vi "agilent test 13.0 Final.vi"() -> ()   [LabVIEW 2023]
uses:
  <vilib>/Utility/file.llb/Write Delimited Spreadsheet (string).vi
  <vilib>/Utility/file.llb/Write Delimited Spreadsheet (DBL).vi
  <vilib>/express/express arith-compare/Formula/XNode/ExpressFormulaBlockNode.xnode
panel:
  in  "Stop running transfer characteristics":bool
  in  "stop OUTPUT":bool
  out "dID":dbl
  in  "SIM VG OUT":dbl[](array[numeric])
  in  "VG OC MEA":dbl[](array[numeric])
  in  "Mobility trans":dbl[](array[numeric])
  in  "IS OUTPUT":dbl[](array[numeric])
  in  "IG OUTPUT":dbl[](array[numeric])
  in  "ID OUTPUT":dbl[](array[numeric])
  in  "VD OUTPUT":dbl[](array[numeric])
  in  "IG TRANSFER":dbl[](array[numeric])
  in  "IS TRANSFER":dbl[](array[numeric])
  in  "ID TRANSFER":dbl[](array[numeric])
  in  "VG TRANSFER":dbl[](array[numeric])
  in  "state":dbl
  in  "output number of times":dbl
  in  "output TEM":dbl
  in  "IDS 6":dbl[](array[numeric])
  in  "IDS 5":dbl[](array[numeric])
  in  "IDS 4":dbl[](array[numeric])
  in  "IDS 3":dbl[](array[numeric])
  in  "IDS 2":dbl[](array[numeric])
  in  "IDS 1":dbl[](array[numeric])
  in  "VDS":dbl[](array[numeric])
  in  "transfer number of times":dbl
  in  "transfer Tem":dbl
  in  "IDS":dbl[](array[numeric])
  in  "VG":dbl[](array[numeric])
  in  "Characterization of TFT":enum32{"Simulation", " Transfer", "Output"}(tab)=enum." Transfer"
  in  "Clear":bool
  in  "Predicted mobility [cm^2/Vs] for OC":dbl
  out "Output characteristic simulation":cluster{"Value":dbl[], "Value":dbl[]}[](graph)
  in  "RUN OUTPUT":bool
  in  "VGS[5] [V] for OC":dbl
  in  "VGS[4] [V] for OC":dbl
  in  "VGS[3] [V] for OC":dbl
  in  "VGS[2] [V] for OC":dbl
  in  "VT [V] for OC":dbl
  in  "VGS[1] [V] for OC":dbl
  in  "Step for VDS [V] for OC":dbl
  in  "Transistor capacitance [nF/cm^2] for OC":dbl
  in  "Transistor length [cm] for OC":dbl
  in  "Transistor width [cm] for OC":dbl
  out "Transfer characteristic simulation":cluster{"Y":dbl[], "Y":dbl[]}[](graph)
  in  "Predicted mobility [cm^2/Vs] for TC":dbl
  in  "Step for VGS [V] for TC":dbl
  in  "Maximum VDS [V] for OC":dbl
  in  "VT [V] for TC":dbl
  in  "VGS [V] for TC":dbl
  in  "Transistor capacitance [nF/cm^2] for TC":dbl
  in  "Transistor width [cm] for TC":dbl
  in  "Transistor length [cm] for TC":dbl
  in  "run":bool
  in  "VG[6] [V] for OC":dbl
  in  "Number of time of hysteresis (TC)":dbl=1.0
  in  "Sample(TC)":dbl=1.0
  out "Mobility":cluster{"Y":dbl[], "Y":dbl[]}[](graph)
  in  "Saturation":bool
  out "Mobility [cm^2/Vs]":dbl
  in  "Hysteresis(TC)":bool
  out "IG/VG":cluster{"Y":dbl[], "Y":dbl[]}[](graph)
  in  "integration(TC)":dbl=1.0
  out "IS/VG":cluster{"Y":dbl[], "Y":dbl[]}[](graph)
  out "ID/VG":cluster{"Y":dbl[], "Y":dbl[]}[](graph)
  out "ID [A](TC)":dbl
  out "IS [A](TC)":dbl
  out "IG [A](TC)":dbl
  in  "Run transfer":bool
  in  "VG Compliance(TC) [A]":dbl=0.001
  in  "VG SMU (T)":dbl=1.0
  in  "VG [V] Step(TC)":dbl=0.01
  in  "VG [V] Stop(TC)":dbl=2.2
  in  "VG [V] Start(TC)":dbl
  in  "VD Compliance(TC) [A] Compliance(TC)":dbl=0.001
  in  "VD SMU (T)":dbl=2.0
  in  "VD [V](TC)":dbl=2.2
  in  "VS Compliance(TC) [A]":dbl=0.001
  in  "VS SMU (T)":dbl=3.0
  in  "VS [V](TC)":dbl
  in  "VISA resource name(TC)":refnum<visa-resource-name>="GPIB0::16::INSTR"
  out "Current VG [V](TC)":dbl
  in  "Length [um]":dbl=10.0
  in  "Thickness [cm]":dbl=3e-07
  in  "Width [um]":dbl=1000.0
  in  "Number of time of hysteresis (OC)":dbl=1.0
  out "VG Measurement number":dbl
  out "VD Measurement number":dbl
  in  "Sample(OC)":dbl=1.0
  out "Current VG [V](OC)":dbl
  in  "Hysteresis(OC)":bool
  out "IG/VD":cluster{"Y":dbl[], "Y":dbl[]}[](graph)
  out "IS/VD":cluster{"Y":dbl[], "Y":dbl[]}[](graph)
  out "ID/VD":cluster{"Y":dbl[], "Y":dbl[]}[](graph)
  out "ID [A](OC)":dbl
  out "IS [A](OC)":dbl
  out "IG [A](OC)":dbl
  in  "VG Compliance(OC) [A]":dbl=0.001
  in  "VG SMU(OC)":dbl=1.0
  out "Current VD [V](OC)":dbl
  in  "VG [V] Step(OC)":dbl=0.4
  in  "VG [V] Stop(OC)":dbl=2.0
  in  "VG [V] Start(OC)":dbl
  in  "VD Compliance(OC) [A]":dbl=0.001
  in  "VD SMU(OC)":dbl=3.0
  in  "VD [V] Step(OC)":dbl=0.01
  in  "VD [V] Stop(OC)":dbl=2.0
  in  "VD [V] Start(OC)":dbl
  in  "VS Compliance(OC) [A]":dbl=0.001
  in  "VS SMU(OC)":dbl=2.0
  in  "VS [V](OC)":dbl
  in  "integration(OC)":dbl=1.0
  in  "RUN OUTPUT":bool
  in  "VISA resource name(OC)":refnum<visa-resource-name>="GPIB0::16::INSTR"
  # "Variables used in program"
  # "Transfer characteristics(TC)"
  # "Please set values below for transfer characteristic simulation"
  # "Run transfer characteristic simulation"
  # "When saving data to file, use .csv as extension filename."
  # "------------------------------------------------------------------------------------------------------------------------------------------------------------------------------------------------------------------------------------------------------------------------------------------------"
  # "Output characteristics(OC)"
  # "Please set values below for output characteristic simulation"
  # "Run output characteristic simulation"
  # "Please press clear to clear data and graph after each run."
  # "This can avoid lag of program"
  # "Clear both graph"
  # "TC stands for transfer characterization"
  # "Linear"
  # "When saving data to file, use .csv as extension filename."
  # "OC stands for output characterization"
  # "When saving data to file, use .csv as extension filename."
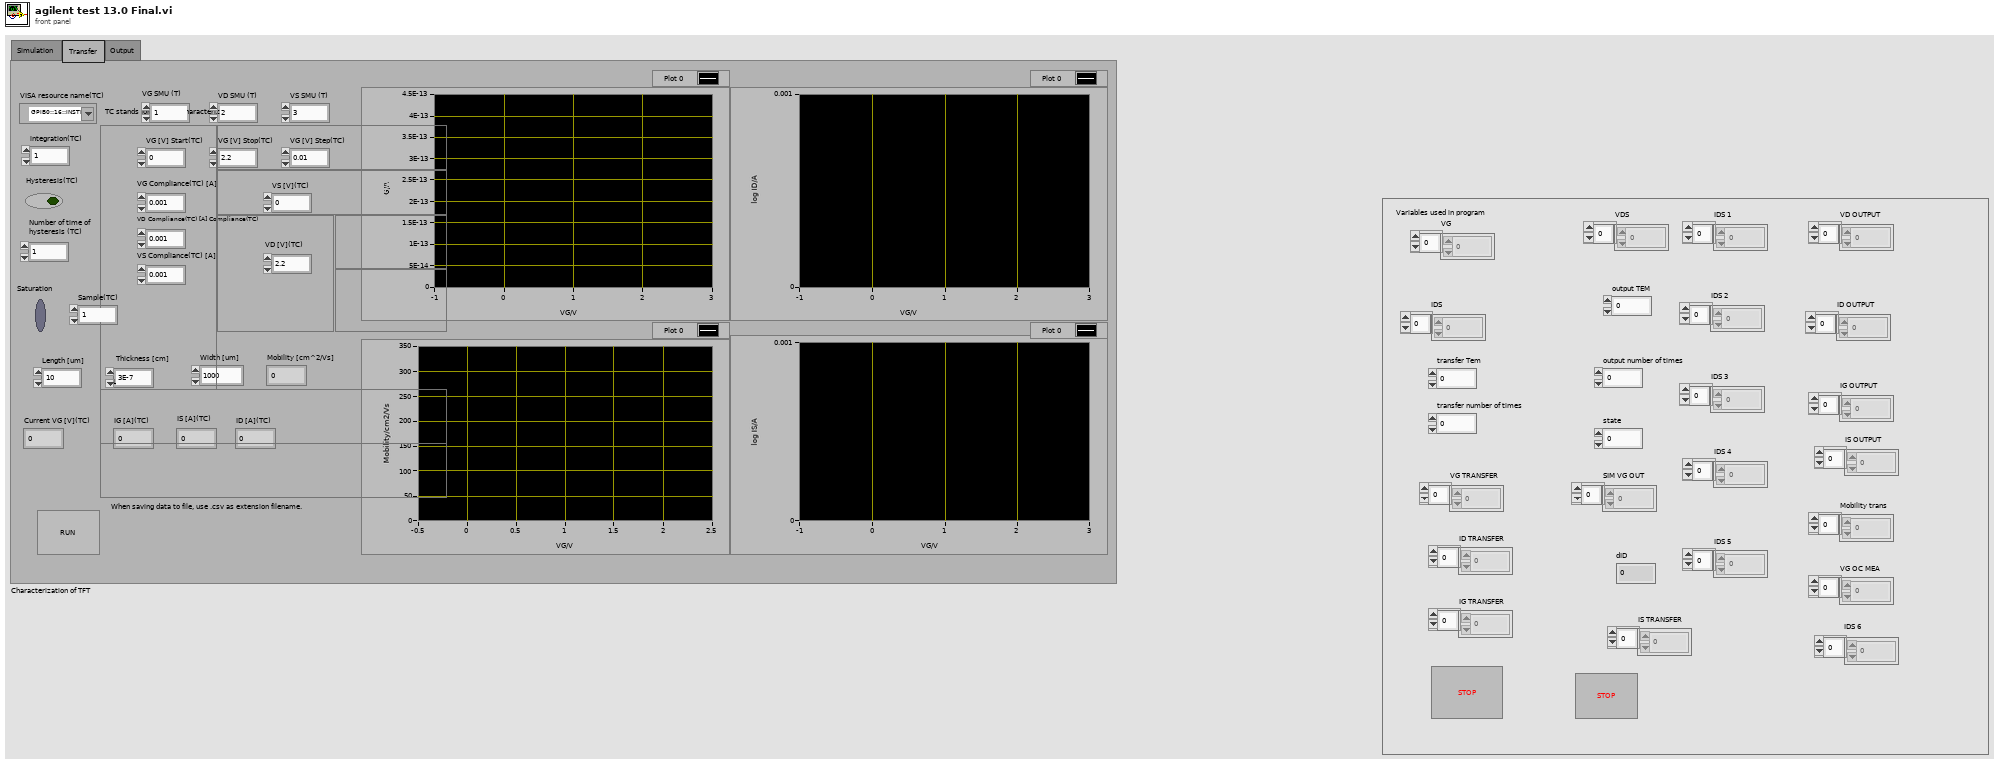
[diagram p1: front panel]
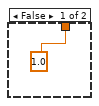
[diagram p3: hidden frame]
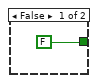
[diagram p4: hidden frame]
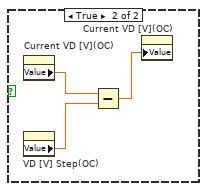
[diagram p5: hidden frame]
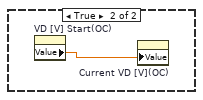
[diagram p6: hidden frame]
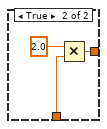
[diagram p7: hidden frame]
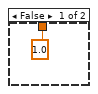
[diagram p10: hidden frame]
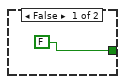
[diagram p12: hidden frame]
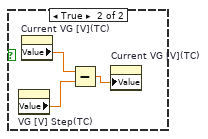
[diagram p13: hidden frame]
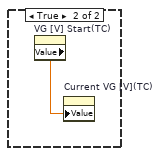
[diagram p14: hidden frame]
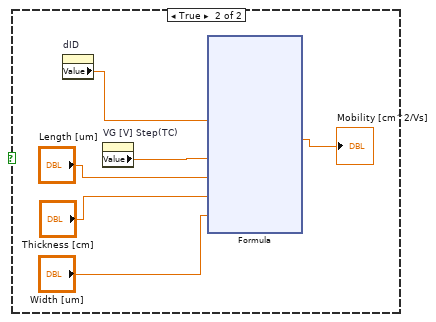
[diagram p15: hidden frame]
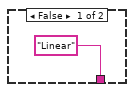
[diagram p17: hidden frame]
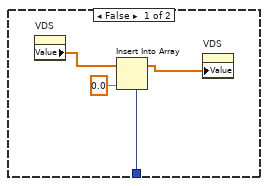
[diagram p18: hidden frame]
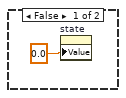
[diagram p19: hidden frame]
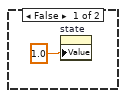
[diagram p20: hidden frame]
diagram:
  n1 = while {
    stop <- FALSE stop-if-true
    n2 = event shown="[0] \"Run transfer\": Value Change" {
      selector: _ -> [_]
      dyn-events: _ -> [_]
      timeout: _ -> [_]
      event "Run transfer": Value Change {
        n3 = event-data() -> ()  [unwired: 1 in, 6 out]
        n4 = while {
          stop <- w6 stop-if-true
          n5 = flat-sequence {
            tunnel: [w12] -> w7
            tunnel: w7 -> [w34]
            tunnel: ["Hysteresis(TC)"] -> w3
            tunnel: [w35] -> w2
            tunnel: [w41] -> w4
            tunnel: w3 -> [w40]
            tunnel: w2 -> [w39]
            tunnel: [TRUE] -> w5
            frame #0 {
              n6 = invoke on="VG TRANSFER" class="Arr (strict)" method="Reinit To Default"() -> ()  [unwired: 3 in, 3 out]
              n7 = invoke on="Mobility trans" class="Arr (strict)" method="Reinit To Default"() -> ()  [unwired: 3 in, 3 out]
              n8 = invoke on="ID TRANSFER" class="Arr (strict)" method="Reinit To Default"() -> ()  [unwired: 3 in, 3 out]
              n9 = property on="Mobility [cm^2/Vs]" class="DigNum (strict)" props=["Value"]() -> ()  [unwired: 2 in, 3 out]
              n10 = invoke on="IG TRANSFER" class="Arr (strict)" method="Reinit To Default"() -> ()  [unwired: 3 in, 3 out]
              n11 = invoke on="IS TRANSFER" class="Arr (strict)" method="Reinit To Default"() -> ()  [unwired: 3 in, 3 out]
              n12 = property on="dID" class="DigNum (strict)"("Value"=0.0 ("dID")) -> ()  [unwired: 2 in, 2 out]
              "Current VG [V](TC)" <- 0.0 ("Transfer tem value")
            }
            frame #1 {
              n13 = Concatenate Strings("*RST", "\n") -> (w23:string)
              n14 = Format Into String(format string="AIT 1,2,%d", "integration(TC)") -> (resulting string=w17:string)  [unwired: 2 in, 1 out]
              n15 = VISA Write(VISA resource name="VISA resource name(TC)", write buffer=w23) -> (VISA resource name out=w22:refnum<visa-resource-name>)  [unwired: 1 in, 2 out]
              n16 = Concatenate Strings(w17, "\n") -> (w14:string)
              n17 = Concatenate Strings("CN;FMT 12,0;AAD 1,1;AAD 2,1;AAD 3,1", "\n") -> (w19:string)
              n18 = VISA Write(VISA resource name=w22, write buffer=w19) -> (VISA resource name out=w13:refnum<visa-resource-name>)  [unwired: 1 in, 2 out]
              n19 = VISA Write(VISA resource name=w13, write buffer=w14) -> (VISA resource name out=w12:refnum<visa-resource-name>)  [unwired: 1 in, 2 out]
            }
            frame #2 {
              n20 = call "Set.vi"("Compliance"="VD Compliance(TC) [A] Compliance(TC)", "Voltage"="VS [V](TC)", "SMU"="VS SMU (T)", "VISA Refnum in"=w34) -> ("VISA Refnum out"=w33:refnum<visa-resource-name>)  [unwired: 7 in]
              n21 = call "Set.vi"("Compliance"="VS Compliance(TC) [A]", "Voltage"="VD [V](TC)", "SMU"="VD SMU (T)", "VISA Refnum in"=w33) -> ()  [unwired: 7 in, 1 out]
            }
            frame #3 {
              n22 = case shown="True" "Hysteresis(TC)" {
                tunnel: [1.0 ("Number of time of hysteresis (TC)") "Number of time of hysteresis (TC)"] -> w35
                frame False {
                }
                frame True {
                }
              }
            }
            frame #4 {
              n23 = for {
                N: w39 -> [_]
                tunnel: [w43] -> w41
                tunnel: w40 -> [w42]
                n24 = flat-sequence {
                  tunnel: [w45] -> w43
                  tunnel: w42 -> [w44]
                  frame #0 {
                    n25 = Subtract(x="VG [V] Stop(TC)", y="VG [V] Start(TC)") -> (x-y=w50:dbl)
                    n26 = Divide(x=w50, y="VG [V] Step(TC)") -> (x/y=w46:dbl)
                    n27 = case shown="True" w44 {
                      tunnel: w46 -> [w53 w56]
                      tunnel: [w53 w54] -> w47
                      frame False {
                      }
                      frame True {
                        n28 = Multiply(x=2.0, y=w56) -> (x*y=w54:dbl)
                      }
                    }
                    n29 = Increment(x=w47) -> (x+1=w48:dbl)
                    n30 = for {
                      N: w48 -> [_]
                      tunnel: w46 -> [w60]
                      tunnel: w44 -> [w58]
                      tunnel: ["Stop running transfer characteristics"] -> w45
                      i -> [w59]
                      stop <- "Stop running transfer characteristics" stop-if-true
                      n31 = flat-sequence {
                        tunnel: w60 -> [w67]
                        tunnel: w59 -> [w66]
                        tunnel: w58 -> [w65]
                        tunnel: ["VG SMU (T)"] -> w64
                        tunnel: [w85] -> w63
                        tunnel: w64 -> [w92]
                        tunnel: w63 -> [w90]
                        tunnel: [w89] -> w62
                        tunnel: w62 -> [w96]
                        tunnel: [w93] -> w61
                        tunnel: w61 -> [w98]
                        frame #0 {
                          n32 = Equal To 0?(x=w66) -> (x = 0?=w68:bool)
                          n33 = case shown="False" w68 {
                            tunnel: w67 -> [w72 _]
                            tunnel: w66 -> [w71 _]
                            tunnel: w65 -> [w69 _]
                            frame False {
                              n34 = case shown="True" w69 {
                                tunnel: w72 -> [_ w76]
                                tunnel: w71 -> [_ w74]
                                tunnel: [FALSE w75] -> w70
                                frame False {
                                }
                                frame True {
                                n35 = Greater?(x=w74, y=w76) -> (0:w75:bool)
                                }
                              }
                              n36 = case shown="False" w70 {
                                frame False {
                                n37 = property on="Current VG [V](TC)" class="DigNum (strict)"() -> ("Value"=w77:dbl)  [unwired: 2 in, 2 out]
                                n38 = property on="VG [V] Step(TC)" class="DigNum (strict)"() -> ("Value"=w78:dbl)  [unwired: 2 in, 2 out]
                                n39 = Add(x=w77, y=w78) -> (x+y=w79:dbl)
                                n40 = property on="Current VG [V](TC)" class="DigNum (strict)"("Value"=w79) -> ()  [unwired: 2 in, 2 out]
                                }
                                frame True {
                                n41 = property on="VG [V] Step(TC)" class="DigNum (strict)"() -> ("Value"=w81:dbl)  [unwired: 2 in, 2 out]
                                n42 = property on="Current VG [V](TC)" class="DigNum (strict)"() -> ("Value"=w82:dbl)  [unwired: 2 in, 2 out]
                                n43 = Subtract(x=w82, y=w81) -> (x-y=w80:dbl)
                                n44 = property on="Current VG [V](TC)" class="DigNum (strict)"("Value"=w80) -> ()  [unwired: 2 in, 2 out]
                                }
                              }
                            }
                            frame True {
                              n45 = property on="VG [V] Start(TC)" class="DigNum (strict)"() -> ("Value"=w83:dbl)  [unwired: 2 in, 2 out]
                              n46 = property on="Current VG [V](TC)" class="DigNum (strict)"("Value"=w83) -> ()  [unwired: 2 in, 2 out]
                            }
                          }
                        }
                        frame #1 {
                          n47 = property on="Current VG [V](TC)" class="DigNum (strict)"() -> ("Value"=w88:dbl)  [unwired: 2 in, 2 out]
                          n48 = property on="VISA resource name(TC)" class="VISAName"() -> ("Value"=w84:refnum<visa-resource-name>)  [unwired: 2 in, 2 out]
                          n49 = call "Set.vi"("Compliance"="VG Compliance(TC) [A]", "Voltage"=w88, "SMU"="VG SMU (T)", "VISA Refnum in"=w84) -> ("VISA Refnum out"=w85:refnum<visa-resource-name>)  [unwired: 7 in]
                        }
                        frame #2 {
                          n50 = call "Read.vi"("SMU"=w92, "VISA Refnum in"=w90) -> ("Current"=→"IG [A](TC)":dbl, "VISA Refnum out"=w89:refnum<visa-resource-name>)  [unwired: 8 in]
                        }
                        frame #3 {
                          n51 = property on="VS SMU (T)" class="DigNum (strict)"() -> ("Value"=w95:dbl)  [unwired: 2 in, 2 out]
                          n52 = call "Read.vi"("SMU"=w95, "VISA Refnum in"=w96) -> ("Current"=→"IS [A](TC)":dbl, "VISA Refnum out"=w93:refnum<visa-resource-name>)  [unwired: 8 in]
                        }
                        frame #4 {
                          n53 = property on="VD SMU (T)" class="DigNum (strict)"() -> ("Value"=w97:dbl)  [unwired: 2 in, 2 out]
                          n54 = call "Read.vi"("SMU"=w97, "VISA Refnum in"=w98) -> ("Current"=→"ID [A](TC)":dbl)  [unwired: 8 in, 1 out]
                        }
                        frame #5 {
                          n55 = property on="IG [A](TC)" class="DigNum (strict)"() -> ("Value"=w109:dbl)  [unwired: 2 in, 2 out]
                          n56 = property on="Current VG [V](TC)" class="DigNum (strict)"() -> ("Value"=w100:dbl)  [unwired: 2 in, 2 out]
                          n57 = Absolute Value(x=w109) -> (abs(x)=w110:dbl)
                          n58 = Build Array (concatenate)("VG TRANSFER", w100) -> (w101:dbl[])
                          n59 = Build Array (concatenate)("IG TRANSFER", w110) -> (w104:dbl[])
                          n60 = property on="VG TRANSFER" class="Arr (strict)"("Value"=w101) -> ()  [unwired: 2 in, 2 out]
                          n61 = property on="IG TRANSFER" class="Arr (strict)"("Value"=w104) -> ()  [unwired: 2 in, 2 out]
                          n62 = property on="IS [A](TC)" class="DigNum (strict)"() -> ("Value"=w111:dbl)  [unwired: 2 in, 2 out]
                          n63 = property on="ID [A](TC)" class="DigNum (strict)"() -> ("Value"=w113:dbl)  [unwired: 2 in, 2 out]
                          n64 = Absolute Value(x=w111) -> (abs(x)=w112:dbl)
                          n65 = Build Array (concatenate)("IS TRANSFER", w112) -> (w106:dbl[])
                          n66 = Absolute Value(x=w113) -> (abs(x)=w114:dbl)
                          n67 = Build Array (concatenate)("ID TRANSFER", w114) -> (w108:dbl[])
                          n68 = property on="ID TRANSFER" class="Arr (strict)"("Value"=w108) -> ()  [unwired: 2 in, 2 out]
                          n69 = property on="IS TRANSFER" class="Arr (strict)"("Value"=w106) -> ()  [unwired: 2 in, 2 out]
                        }
                        frame #6 {
                          n70 = property on="ID TRANSFER" class="Arr (strict)"() -> ("Value"=w123:dbl[])  [unwired: 2 in, 2 out]
                          n71 = Array Size(array=w123) -> (size(s)=w116:i32)
                          n72 = Decrement(x=w116) -> (x-1=w115:i32)
                          n73 = Decrement(x=w115) -> (x-1=w122:i32)
                          n74 = Index Array(array=w123, index=w122) -> (element=w125:dbl)
                          n75 = Absolute Value(x=w125) -> (abs(x)=w119:dbl)
                          n76 = property on="ID [A](TC)" class="DigNum (strict)"() -> ("Value"=w124:dbl)  [unwired: 2 in, 2 out]
                          n77 = Absolute Value(x=w124) -> (abs(x)=w120:dbl)
                          n78 = Subtract(x=w120, y=w119) -> (x-y=w121:dbl)
                          n79 = Absolute Value(x=w121) -> (abs(x)=w118:dbl)
                          n80 = Square Root(x=w118) -> (sqrt(x)=→"dID":dbl)
                        }
                        frame #7 {
                          n81 = case shown="False" "Saturation" {
                            frame False {
                              n82 = property on="VG [V] Step(TC)" class="DigNum (strict)"() -> ("Value"=w129:dbl)  [unwired: 2 in, 2 out]
                              n83 = property on="dID" class="DigNum (strict)"() -> ("Value"=w127:dbl)  [unwired: 2 in, 2 out]
                              n84 = property on="VD [V](TC)" class="DigNum (strict)"() -> ("Value"=w130:dbl)  [unwired: 2 in, 2 out]
                              n85 = property on="Length [um]" class="DigNum (strict)"() -> ("Value"=w133:dbl)  [unwired: 2 in, 2 out]
                              n86 = property on="Thickness [cm]" class="DigNum (strict)"() -> ("Value"=w132:dbl)  [unwired: 2 in, 2 out]
                              n87 = property on="Width [um]" class="DigNum (strict)"() -> ("Value"=w131:dbl)  [unwired: 2 in, 2 out]
                              n88 = xnode "Formula"("dID"=w127, "dVG"=w129, "L"=w133, "t"=w132, "VD"=w130, "W"=w131) -> ("Result"=w128:dbl)  [unwired: 1 in, 1 out]
                              n89 = property on="Mobility [cm^2/Vs]" class="DigNum (strict)"("Value"=w128) -> ()  [unwired: 2 in, 2 out]
                            }
                            frame True {
                              n90 = property on="dID" class="DigNum (strict)"() -> ("Value"=w152:dbl)  [unwired: 2 in, 2 out]
                              n91 = property on="VG [V] Step(TC)" class="DigNum (strict)"() -> ("Value"=w153:dbl)  [unwired: 2 in, 2 out]
                              n92 = xnode "Formula"("dID"=w152, "dVG"=w153, "L"="Length [um]", "t"="Thickness [cm]", "W"="Width [um]") -> ("Result"=→"Mobility [cm^2/Vs]":dbl)  [unwired: 1 in, 1 out]
                            }
                          }
                        }
                        frame #8 {
                          n93 = property on="Mobility [cm^2/Vs]" class="DigNum (strict)"() -> ("Value"=w176:dbl)  [unwired: 2 in, 2 out]
                          n94 = Absolute Value(x=w176) -> (abs(x)=w177:dbl)
                          n95 = Build Array (concatenate)("Mobility trans", w177) -> (w175:dbl[])
                          n96 = property on="Mobility trans" class="Arr (strict)"("Value"=w175) -> ()  [unwired: 2 in, 2 out]
                        }
                        frame #9 {
                          n97 = property on="Mobility trans" class="Arr (strict)"() -> ("Value"=w183:dbl[])  [unwired: 2 in, 2 out]
                          n98 = property on="IS TRANSFER" class="Arr (strict)"() -> ("Value"=w195:dbl[])  [unwired: 2 in, 2 out]
                          n99 = property on="IG TRANSFER" class="Arr (strict)"() -> ("Value"=w186:dbl[])  [unwired: 2 in, 2 out]
                          n100 = property on="VG TRANSFER" class="Arr (strict)"() -> ("Value"=w178:dbl[])  [unwired: 2 in, 2 out]
                          n101 = property on="ID TRANSFER" class="Arr (strict)"() -> ("Value"=w194:dbl[])  [unwired: 2 in, 2 out]
                          n102 = Absolute Value(x=w183) -> (abs(x)=w182:dbl[])
                          n103 = Absolute Value(x=w194) -> (abs(x)=w193:dbl[])
                          n104 = Absolute Value(x=w195) -> (abs(x)=w192:dbl[])
                          n105 = Absolute Value(x=w186) -> (abs(x)=w187:dbl[])
                          n106 = call "Convert to Dynamic Data8"("Array"=w187) -> ("Dynamic Data Type"=w185:dynamicdata)  [unwired: 3 in]
                          n107 = call "Convert to Dynamic Data6"("Array"=w193) -> ("Dynamic Data Type"=w191:dynamicdata)  [unwired: 3 in]
                          n108 = call "Convert to Dynamic Data13"("Array"=w182) -> ("Dynamic Data Type"=w181:dynamicdata)  [unwired: 3 in]
                          n109 = call "Convert to Dynamic Data5"("Array"=w178) -> ("Dynamic Data Type"=w180:dynamicdata)  [unwired: 3 in]
                          n110 = call "Convert to Dynamic Data7"("Array"=w192) -> ("Dynamic Data Type"=w190:dynamicdata)  [unwired: 3 in]
                          n111 = call "IS3"("Y Input"=w185, "X Input"=w180) -> ("XY Graph"=→"IG/VG":cluster{"Y":dbl[], "Y":dbl[]}[])  [unwired: 3 in, 6 out]
                          n112 = call "IS7"("Y Input"=w181, "X Input"=w180) -> ("XY Graph"=→"Mobility":cluster{"Y":dbl[], "Y":dbl[]}[])  [unwired: 3 in, 6 out]
                          n113 = call "IS"("Y Input"=w191, "X Input"=w180) -> ("XY Graph"=→"ID/VG":cluster{"Y":dbl[], "Y":dbl[]}[])  [unwired: 3 in, 6 out]
                          n114 = call "IS2"("Y Input"=w190, "X Input"=w180) -> ("XY Graph"=→"IS/VG":cluster{"Y":dbl[], "Y":dbl[]}[])  [unwired: 3 in, 6 out]
                        }
                      }
                    }
                  }
                  frame #1 {
                    n115 = property on="Current VG [V](TC)" class="DigNum (strict)"("Value"=0.0 ("Current VG [V](TC)")) -> ()  [unwired: 2 in, 2 out]
                  }
                }
              }
            }
            frame #5 {
              n116 = flat-sequence {
                tunnel: [w198] -> w197
                tunnel: w197 -> [w209]
                frame #0 {
                  w199 = 0.0001 ("Compliance")
                  n117 = property on="VISA resource name(TC)" class="VISAName"() -> ("Value"=w208:refnum<visa-resource-name>)  [unwired: 2 in, 2 out]
                  n118 = call "Set.vi"("Compliance"=w199, "Voltage"=0.0, "SMU"=1.0, "VISA Refnum in"=w208) -> ("VISA Refnum out"=w207:refnum<visa-resource-name>)  [unwired: 7 in]
                  n119 = call "Set.vi"("Compliance"=w199, "Voltage"=0.0, "SMU"=2.0, "VISA Refnum in"=w207) -> ("VISA Refnum out"=w206:refnum<visa-resource-name>)  [unwired: 7 in]
                  n120 = call "Set.vi"("Compliance"=w199, "Voltage"=0.0, "SMU"=3.0, "VISA Refnum in"=w206) -> ("VISA Refnum out"=w198:refnum<visa-resource-name>)  [unwired: 7 in]
                }
                frame #1 {
                  n121 = Concatenate Strings("*RST; DZ;CL", "\n") -> (w210:string)
                  n122 = VISA Write(VISA resource name=w209, write buffer=w210) -> ()  [unwired: 1 in, 3 out]
                }
              }
            }
            frame #6 {
              n123 = Two Button Dialog(message="Do you want to save data? (If save, please save as .csv)", 1:"Don't save" ("F button name (\"Cancel\")"), 2:"Save" ("T button name (\"OK\")")) -> (T button?=w216:bool)
              n124 = case shown="True" w216 {
                frame False {
                }
                frame True {
                  n125 = flat-sequence {
                    tunnel: [w225] -> w218
                    tunnel: [w229] -> w219
                    tunnel: w218 -> [w228]
                    tunnel: [w236] -> w221
                    tunnel: w219 -> [w235]
                    tunnel: w221 -> [w258]
                    tunnel: [w244] -> w220
                    tunnel: w220 -> [w265]
                    tunnel: [w263] -> w217
                    tunnel: w217 -> [w276]
                    frame #0 {
                      n126 = call-poly <vilib>:"Write Delimited Spreadsheet.vi"("1D data"=string[] ["Date", "Time"], "append to file? (new file:F)"=TRUE, "delimiter (\\t)"="," ("delimiter (\\t)")) -> ("new file path (Not A Path if cancelled)"=w225:path)  [unwired: 11 in, 1 out]
                    }
                    frame #1 {
                      n127 = Get Date/Time String() -> (date string=w232:string, time string=w231:string)  [unwired: 1 in, 2 out]
                      n128 = Build Array(w232, w231) -> (w230:string[])
                      n129 = call-poly <vilib>:"Write Delimited Spreadsheet.vi"("file path (dialog if empty)"=w228, "1D data"=w230, "append to file? (new file:F)"=TRUE, "delimiter (\\t)"="," ("delimiter (\\t)")) -> ("new file path (Not A Path if cancelled)"=w229:path)  [unwired: 10 in, 1 out]
                    }
                    frame #2 {
                      n130 = call-poly <vilib>:"Write Delimited Spreadsheet.vi"("file path (dialog if empty)"=w235, "1D data"=string[] ["Sample", "Integration", "Thickness/cm", "Width/cm", "Length/cm", "Regime", "VS/V", "VD/V"], "append to file? (new file:F)"=TRUE, "delimiter (\\t)"="," ("delimiter (\\t)")) -> ("new file path (Not A Path if cancelled)"=w236:path)  [unwired: 10 in, 1 out]
                    }
                    frame #3 {
                      n131 = property on="integration(TC)" class="DigNum (strict)"() -> ("Value"=w256:dbl)  [unwired: 2 in, 2 out]
                      n132 = property on="Thickness [cm]" class="DigNum (strict)"() -> ("Value"=w255:dbl)  [unwired: 2 in, 2 out]
                      n133 = property on="Saturation" class="Bool (strict)"() -> ("Value"=w239:bool)  [unwired: 2 in, 2 out]
                      n134 = property on="Width [um]" class="DigNum (strict)"() -> ("Value"=w254:dbl)  [unwired: 2 in, 2 out]
                      n135 = property on="Length [um]" class="DigNum (strict)"() -> ("Value"=w253:dbl)  [unwired: 2 in, 2 out]
                      n136 = Number To Decimal String(number="Sample(TC)") -> (decimal integer string=w252:string)  [unwired: 1 out]
                      n137 = Number To Decimal String(number=w253) -> (decimal integer string=w248:string)  [unwired: 1 out]
                      n138 = Number To Decimal String(number=w256) -> (decimal integer string=w251:string)  [unwired: 1 out]
                      n139 = Number To Decimal String(number=w254) -> (decimal integer string=w249:string)  [unwired: 1 out]
                      n140 = Number To Decimal String(number=w255) -> (decimal integer string=w250:string)  [unwired: 1 out]
                      n141 = case shown="True" w239 {
                        tunnel: ["Linear" "Saturation"] -> w247
                        frame False {
                        }
                        frame True {
                        }
                      }
                      n142 = property on="VS [V](TC)" class="DigNum (strict)"() -> ("Value"=w243:dbl)  [unwired: 2 in, 2 out]
                      n143 = property on="VD [V](TC)" class="DigNum (strict)"() -> ("Value"=w242:dbl)  [unwired: 2 in, 2 out]
                      n144 = Number To Decimal String(number=w243) -> (decimal integer string=w241:string)  [unwired: 1 out]
                      n145 = Number To Decimal String(number=w242) -> (decimal integer string=w240:string)  [unwired: 1 out]
                      n146 = Build Array(w252, w251, w250, w249, w248, w247, w241, w240) -> (w246:string[])
                      n147 = call-poly <vilib>:"Write Delimited Spreadsheet.vi"("file path (dialog if empty)"=w258, "1D data"=w246, "append to file? (new file:F)"=TRUE, "delimiter (\\t)"="," ("delimiter (\\t)")) -> ("new file path (Not A Path if cancelled)"=w244:path)  [unwired: 10 in, 1 out]
                    }
                    frame #4 {
                      n148 = call-poly <vilib>:"Write Delimited Spreadsheet.vi"("file path (dialog if empty)"=w265, "1D data"=string[] ["VG/V", "IG/A", "IS/A", "ID/A", "Mobility/cm^2/Vs"], "append to file? (new file:F)"=TRUE, "delimiter (\\t)"="," ("delimiter (\\t)")) -> ("new file path (Not A Path if cancelled)"=w263:path)  [unwired: 10 in, 1 out]
                    }
                    frame #5 {
                      n149 = property on="VG TRANSFER" class="Arr (strict)"() -> ("Value"=w275:dbl[])  [unwired: 2 in, 2 out]
                      n150 = property on="IG TRANSFER" class="Arr (strict)"() -> ("Value"=w274:dbl[])  [unwired: 2 in, 2 out]
                      n151 = property on="IS TRANSFER" class="Arr (strict)"() -> ("Value"=w273:dbl[])  [unwired: 2 in, 2 out]
                      n152 = property on="ID TRANSFER" class="Arr (strict)"() -> ("Value"=w272:dbl[])  [unwired: 2 in, 2 out]
                      n153 = property on="Mobility trans" class="Arr (strict)"() -> ("Value"=w271:dbl[])  [unwired: 2 in, 2 out]
                      n154 = Build Array(w275, w274, w273, w272, w271) -> (w270:dbl[][])
                      n155 = call-poly <vilib>:"Write Delimited Spreadsheet.vi"("file path (dialog if empty)"=w276, "format (%.3f)"="%.5e", "2D data"=w270, "append to file? (new file:F)"=TRUE, "transpose? (no:F)"=TRUE, "delimiter (\\t)"="," ("delimiter (\\t)")) -> ()  [unwired: 8 in, 2 out]
                    }
                  }
                }
              }
            }
            frame #7 {
            }
          }
          n156 = case shown="True" w4 {
            selector: w4 -> [_ w9]
            tunnel: [w8 w9] -> w6
            tunnel: w5 -> [w8 _]
            frame False {
            }
            frame True {
            }
          }
        }
      }
    }
  }
  n157 = while {
    stop <- FALSE stop-if-true
    n158 = event shown="[0] \"RUN OUTPUT\": Value Change" {
      selector: _ -> [_]
      dyn-events: _ -> [_]
      timeout: _ -> [_]
      event "RUN OUTPUT": Value Change {
        n159 = event-data() -> ()  [unwired: 1 in, 6 out]
        n160 = while {
          stop <- w283 stop-if-true
          n161 = flat-sequence {
            tunnel: [w290] -> w284
            tunnel: w284 -> [w305]
            tunnel: ["Hysteresis(OC)"] -> w280
            tunnel: [w309] -> w279
            tunnel: [w315] -> w281
            tunnel: w280 -> [w314]
            tunnel: w279 -> [w313]
            tunnel: [TRUE] -> w282
            frame #0 {
              n162 = invoke on="VG OC MEA" class="Arr (strict)" method="Reinit To Default"() -> ()  [unwired: 3 in, 3 out]
              n163 = invoke on="VD OUTPUT" class="Arr (strict)" method="Reinit To Default"() -> ()  [unwired: 3 in, 3 out]
              n164 = invoke on="ID OUTPUT" class="Arr (strict)" method="Reinit To Default"() -> ()  [unwired: 3 in, 3 out]
              n165 = invoke on="IG OUTPUT" class="Arr (strict)" method="Reinit To Default"() -> ()  [unwired: 3 in, 3 out]
              n166 = invoke on="IS OUTPUT" class="Arr (strict)" method="Reinit To Default"() -> ()  [unwired: 3 in, 3 out]
              "Current VD [V](OC)" <- 0.0 ("Current VD(OC)")
              "VD Measurement number" <- 0.0 ("VD Measurement number")
              "VG Measurement number" <- 0.0 ("VG Measurement number")
            }
            frame #1 {
              n167 = Concatenate Strings("*RST", "\n") -> (w300:string)
              n168 = Format Into String(format string="AIT 1,2,%d", "integration(OC)") -> (resulting string=w294:string)  [unwired: 2 in, 1 out]
              n169 = VISA Write(VISA resource name="VISA resource name(OC)", write buffer=w300) -> (VISA resource name out=w298:refnum<visa-resource-name>)  [unwired: 1 in, 2 out]
              n170 = Concatenate Strings("CN;FMT 12,0;AAD 1,1;AAD 2,1;AAD 3,1", "\n") -> (w299:string)
              n171 = VISA Write(VISA resource name=w298, write buffer=w299) -> (VISA resource name out=w296:refnum<visa-resource-name>)  [unwired: 1 in, 2 out]
              n172 = Concatenate Strings(w294, "\n") -> (w291:string)
              n173 = VISA Write(VISA resource name=w296, write buffer=w291) -> (VISA resource name out=w290:refnum<visa-resource-name>)  [unwired: 1 in, 2 out]
            }
            frame #2 {
              n174 = call "Set.vi"("Compliance"="VS Compliance(OC) [A]", "Voltage"="VS [V](OC)", "SMU"="VS SMU(OC)", "VISA Refnum in"=w305) -> ()  [unwired: 7 in, 1 out]
            }
            frame #3 {
              n175 = case shown="True" "Hysteresis(OC)" {
                tunnel: [1.0 ("Number of time of hysteresis (OC)") "Number of time of hysteresis (OC)"] -> w309
                frame False {
                }
                frame True {
                }
              }
            }
            frame #4 {
              n176 = for {
                N: w313 -> [_]
                shift-right: [w317] -> w315
                shift-left: w314 -> [w316]
                n177 = flat-sequence {
                  tunnel: [w321] -> w317
                  tunnel: w316 -> [w320]
                  frame #0 {
                    n178 = Subtract(x="VD [V] Stop(OC)", y="VD [V] Start(OC)") -> (x-y=w330:dbl)
                    n179 = Divide(x=w330, y="VD [V] Step(OC)") -> (x/y=w322:dbl)
                    n180 = property on="VD Measurement number" class="DigNum (strict)"("Value"=w322) -> ()  [unwired: 2 in, 2 out]
                    n181 = case shown="False" w320 {
                      tunnel: w322 -> [w415 w417]
                      tunnel: [w415 w416] -> w328
                      frame False {
                      }
                      frame True {
                        n182 = Multiply(x=2.0, y=w417) -> (x*y=w416:dbl)
                      }
                    }
                    n183 = Subtract(x="VG [V] Stop(OC)", y="VG [V] Start(OC)") -> (x-y=w325:dbl)
                    n184 = Divide(x=w325, y="VG [V] Step(OC)") -> (x/y=w319:dbl)
                    n185 = Increment(x=w319) -> (x+1=w318:dbl)
                    n186 = property on="VG Measurement number" class="DigNum (strict)"("Value"=w318) -> ()  [unwired: 2 in, 2 out]
                    n187 = Increment(x=w328) -> (x+1=w327:dbl)
                    n188 = for {
                      N: w318 -> [_]
                      tunnel: w327 -> [w339]
                      tunnel: w322 -> [w338]
                      tunnel: w320 -> [w337]
                      shift-right: [w335] -> _
                      shift-left: "VG [V] Start(OC)" -> [w334]
                      tunnel: "VG [V] Step(OC)" -> [w336]
                      tunnel: ["stop OUTPUT"] -> w321
                      stop <- "stop OUTPUT" stop-if-true
                      n189 = property on="VISA resource name(OC)" class="VISAName"() -> ("Value"=w342:refnum<visa-resource-name>)  [unwired: 2 in, 2 out]
                      n190 = Add(x=w334, y=w336) -> (x+y=w335:dbl)
                      n191 = call "Set.vi"("Compliance"="VG Compliance(OC) [A]", "Voltage"=w334, "SMU"="VG SMU(OC)", "VISA Refnum in"=w342) -> ()  [unwired: 7 in, 1 out]
                      n192 = for {
                        N: w339 -> [_]
                        tunnel: w338 -> [w345]
                        tunnel: w337 -> [w344]
                        tunnel: w334 -> [w343]
                        i -> [w350]
                        n193 = flat-sequence {
                          tunnel: w350 -> [w353]
                          tunnel: w345 -> [w352]
                          tunnel: w344 -> [w351]
                          tunnel: [w371] -> w349
                          tunnel: ["VD SMU(OC)"] -> w348
                          tunnel: w349 -> [w378]
                          tunnel: w348 -> [w377]
                          tunnel: [w375] -> w347
                          tunnel: w347 -> [w381]
                          tunnel: [w380] -> w346
                          tunnel: w346 -> [w384]
                          tunnel: w343 -> [w393]
                          frame #0 {
                            n194 = Equal To 0?(x=w353) -> (x = 0?=w354:bool)
                            n195 = case shown="False" w354 {
                              tunnel: w353 -> [w358 _]
                              tunnel: w352 -> [w357 _]
                              tunnel: w351 -> [w355 _]
                              frame False {
                                n196 = case shown="True" w355 {
                                tunnel: w358 -> [_ w360]
                                tunnel: w357 -> [_ w362]
                                tunnel: [FALSE w361] -> w356
                                frame False {
                                }
                                frame True {
                                n197 = Greater?(x=w360, y=w362) -> (0:w361:bool)
                                }
                                }
                                n198 = case shown="False" w356 {
                                frame False {
                                n199 = property on="VD [V] Step(OC)" class="DigNum (strict)"() -> ("Value"=w364:dbl)  [unwired: 2 in, 2 out]
                                n200 = property on="Current VD [V](OC)" class="DigNum (strict)"() -> ("Value"=w363:dbl)  [unwired: 2 in, 2 out]
                                n201 = Add(x=w363, y=w364) -> (x+y=w365:dbl)
                                n202 = property on="Current VD [V](OC)" class="DigNum (strict)"("Value"=w365) -> ()  [unwired: 2 in, 2 out]
                                }
                                frame True {
                                n203 = property on="Current VD [V](OC)" class="DigNum (strict)"() -> ("Value"=w368:dbl)  [unwired: 2 in, 2 out]
                                n204 = property on="VD [V] Step(OC)" class="DigNum (strict)"() -> ("Value"=w367:dbl)  [unwired: 2 in, 2 out]
                                n205 = Subtract(x=w368, y=w367) -> (x-y=w366:dbl)
                                n206 = property on="Current VD [V](OC)" class="DigNum (strict)"("Value"=w366) -> ()  [unwired: 2 in, 2 out]
                                }
                                }
                              }
                              frame True {
                                n207 = property on="VD [V] Start(OC)" class="DigNum (strict)"() -> ("Value"=w369:dbl)  [unwired: 2 in, 2 out]
                                n208 = property on="Current VD [V](OC)" class="DigNum (strict)"("Value"=w369) -> ()  [unwired: 2 in, 2 out]
                              }
                            }
                          }
                          frame #1 {
                            n209 = property on="Current VD [V](OC)" class="DigNum (strict)"() -> ("Value"=w373:dbl)  [unwired: 2 in, 2 out]
                            n210 = property on="VISA resource name(OC)" class="VISAName"() -> ("Value"=w374:refnum<visa-resource-name>)  [unwired: 2 in, 2 out]
                            n211 = call "Set.vi"("Compliance"="VD Compliance(OC) [A]", "Voltage"=w373, "SMU"="VD SMU(OC)", "VISA Refnum in"=w374) -> ("VISA Refnum out"=w371:refnum<visa-resource-name>)  [unwired: 7 in]
                          }
                          frame #2 {
                            n212 = call "Read.vi"("SMU"=w377, "VISA Refnum in"=w378) -> ("Current"=→"ID [A](OC)":dbl, "VISA Refnum out"=w375:refnum<visa-resource-name>)  [unwired: 8 in]
                          }
                          frame #3 {
                            n213 = property on="VS SMU(OC)" class="DigNum (strict)"() -> ("Value"=w379:dbl)  [unwired: 2 in, 2 out]
                            n214 = call "Read.vi"("SMU"=w379, "VISA Refnum in"=w381) -> ("Current"=→"IS [A](OC)":dbl, "VISA Refnum out"=w380:refnum<visa-resource-name>)  [unwired: 8 in]
                          }
                          frame #4 {
                            n215 = property on="VG SMU(OC)" class="DigNum (strict)"() -> ("Value"=w383:dbl)  [unwired: 2 in, 2 out]
                            n216 = call "Read.vi"("SMU"=w383, "VISA Refnum in"=w384) -> ("Current"=→"IG [A](OC)":dbl)  [unwired: 8 in, 1 out]
                          }
                          frame #5 {
                            n217 = property on="Current VD [V](OC)" class="DigNum (strict)"() -> ("Value"=w386:dbl)  [unwired: 2 in, 2 out]
                            n218 = property on="ID [A](OC)" class="DigNum (strict)"() -> ("Value"=w390:dbl)  [unwired: 2 in, 2 out]
                            n219 = Absolute Value(x=w390) -> (abs(x)=w389:dbl)
                            n220 = Build Array (concatenate)("ID OUTPUT", w389) -> (w399:dbl[])
                            n221 = Build Array (concatenate)("VD OUTPUT", w386) -> (w402:dbl[])
                            n222 = property on="ID OUTPUT" class="Arr (strict)"("Value"=w399) -> ()  [unwired: 2 in, 2 out]
                            n223 = Build Array (concatenate)("VG OC MEA", w393) -> (w394:dbl[])
                            n224 = property on="VD OUTPUT" class="Arr (strict)"("Value"=w402) -> ()  [unwired: 2 in, 2 out]
                            n225 = property on="IG [A](OC)" class="DigNum (strict)"() -> ("Value"=w392:dbl)  [unwired: 2 in, 2 out]
                            n226 = property on="IS [A](OC)" class="DigNum (strict)"() -> ("Value"=w388:dbl)  [unwired: 2 in, 2 out]
                            n227 = property on="VG OC MEA" class="Arr (strict)"("Value"=w394) -> ()  [unwired: 2 in, 2 out]
                            n228 = Absolute Value(x=w392) -> (abs(x)=w391:dbl)
                            n229 = Absolute Value(x=w388) -> (abs(x)=w387:dbl)
                            n230 = Build Array (concatenate)("IG OUTPUT", w391) -> (w398:dbl[])
                            n231 = Build Array (concatenate)("IS OUTPUT", w387) -> (w396:dbl[])
                            n232 = property on="IG OUTPUT" class="Arr (strict)"("Value"=w398) -> ()  [unwired: 2 in, 2 out]
                            n233 = property on="IS OUTPUT" class="Arr (strict)"("Value"=w396) -> ()  [unwired: 2 in, 2 out]
                          }
                          frame #6 {
                            n234 = property on="VD OUTPUT" class="Arr (strict)"() -> ("Value"=w414:dbl[])  [unwired: 2 in, 2 out]
                            n235 = property on="IG OUTPUT" class="Arr (strict)"() -> ("Value"=w412:dbl[])  [unwired: 2 in, 2 out]
                            n236 = property on="ID OUTPUT" class="Arr (strict)"() -> ("Value"=w413:dbl[])  [unwired: 2 in, 2 out]
                            n237 = property on="IS OUTPUT" class="Arr (strict)"() -> ("Value"=w411:dbl[])  [unwired: 2 in, 2 out]
                            n238 = call "Convert to Dynamic Data9"("Array"=w414) -> ("Dynamic Data Type"=w410:dynamicdata)  [unwired: 3 in]
                            n239 = call "Convert to Dynamic Data10"("Array"=w413) -> ("Dynamic Data Type"=w409:dynamicdata)  [unwired: 3 in]
                            n240 = call "Convert to Dynamic Data11"("Array"=w412) -> ("Dynamic Data Type"=w407:dynamicdata)  [unwired: 3 in]
                            n241 = call "Convert to Dynamic Data12"("Array"=w411) -> ("Dynamic Data Type"=w405:dynamicdata)  [unwired: 3 in]
                            n242 = call "IS4"("Y Input"=w407, "X Input"=w410) -> ("XY Graph"=→"IG/VD":cluster{"Y":dbl[], "Y":dbl[]}[])  [unwired: 3 in, 6 out]
                            n243 = call "IS5"("Y Input"=w409, "X Input"=w410) -> ("XY Graph"=→"ID/VD":cluster{"Y":dbl[], "Y":dbl[]}[])  [unwired: 3 in, 6 out]
                            n244 = call "IS6"("Y Input"=w405, "X Input"=w410) -> ("XY Graph"=→"IS/VD":cluster{"Y":dbl[], "Y":dbl[]}[])  [unwired: 3 in, 6 out]
                          }
                        }
                      }
                      "Current VG [V](OC)" <- w334
                    }
                  }
                  frame #1 {
                    n245 = property on="Current VD [V](OC)" class="DigNum (strict)"("Value"=0.0 ("Current VD [V](OC)")) -> ()  [unwired: 2 in, 2 out]
                  }
                }
              }
            }
            frame #5 {
              n246 = flat-sequence {
                tunnel: [w426] -> w420
                tunnel: w420 -> [w430]
                frame #0 {
                  w421 = 0.0001 ("Compliance")
                  w422 = 0.0 ("Voltage")
                  n247 = property on="VISA resource name(OC)" class="VISAName"() -> ("Value"=w429:refnum<visa-resource-name>)  [unwired: 2 in, 2 out]
                  n248 = call "Set.vi"("Compliance"=w421, "Voltage"=w422, "SMU"=1.0, "VISA Refnum in"=w429) -> ("VISA Refnum out"=w428:refnum<visa-resource-name>)  [unwired: 7 in]
                  n249 = call "Set.vi"("Compliance"=w421, "Voltage"=w422, "SMU"=2.0, "VISA Refnum in"=w428) -> ("VISA Refnum out"=w427:refnum<visa-resource-name>)  [unwired: 7 in]
                  n250 = call "Set.vi"("Compliance"=w421, "Voltage"=w422, "SMU"=3.0, "VISA Refnum in"=w427) -> ("VISA Refnum out"=w426:refnum<visa-resource-name>)  [unwired: 7 in]
                }
                frame #1 {
                  n251 = Concatenate Strings("*RST; DZ;CL", "\n") -> (w431:string)
                  n252 = VISA Write(VISA resource name=w430, write buffer=w431) -> ()  [unwired: 1 in, 3 out]
                }
              }
            }
            frame #6 {
              n253 = Two Button Dialog(message="Do you want to save data? (If save, please save as .csv)", 1:"Don't save" ("F button name (\"Cancel\")"), 2:"Save" ("T button name (\"OK\")")) -> (T button?=w437:bool)
              n254 = case shown="True" w437 {
                frame False {
                }
                frame True {
                  n255 = flat-sequence {
                    tunnel: [w443] -> w440
                    tunnel: w440 -> [w450]
                    tunnel: [w449] -> w439
                    tunnel: w439 -> [w466]
                    tunnel: [w463] -> w438
                    tunnel: w438 -> [w470]
                    frame #0 {
                      n256 = call-poly <vilib>:"Write Delimited Spreadsheet.vi"("1D data"=string[] ["Date", "Time", "Sample", "Integration", "VS/V", "VD Measurement number", "VG Measurement number"], "append to file? (new file:F)"=TRUE, "delimiter (\\t)"="," ("delimiter (\\t)")) -> ("new file path (Not A Path if cancelled)"=w443:path)  [unwired: 11 in, 1 out]
                    }
                    frame #1 {
                      n257 = Get Date/Time String() -> (date string=w457:string, time string=w456:string)  [unwired: 3 in]
                      n258 = property on="integration(OC)" class="DigNum (strict)"() -> ("Value"=w460:dbl)  [unwired: 2 in, 2 out]
                      n259 = property on="VS [V](OC)" class="DigNum (strict)"() -> ("Value"=w459:dbl)  [unwired: 2 in, 2 out]
                      n260 = property on="VD Measurement number" class="DigNum (strict)"() -> ("Value"=w458:dbl)  [unwired: 2 in, 2 out]
                      n261 = property on="VG Measurement number" class="DigNum (strict)"() -> ("Value"=w446:dbl)  [unwired: 2 in, 2 out]
                      n262 = Number To Decimal String(number=w460) -> (decimal integer string=w454:string)  [unwired: 1 out]
                      n263 = Number To Decimal String(number=w458) -> (decimal integer string=w452:string)  [unwired: 1 out]
                      n264 = Number To Decimal String(number=w459) -> (decimal integer string=w453:string)  [unwired: 1 out]
                      n265 = Number To Decimal String(number="Sample(OC)") -> (decimal integer string=w455:string)  [unwired: 1 out]
                      n266 = Number To Decimal String(number=w446) -> (decimal integer string=w445:string)  [unwired: 1 out]
                      n267 = Build Array(w457, w456, w455, w454, w453, w452, w445) -> (w451:string[])
                      n268 = call-poly <vilib>:"Write Delimited Spreadsheet.vi"("file path (dialog if empty)"=w450, "1D data"=w451, "append to file? (new file:F)"=TRUE, "delimiter (\\t)"="," ("delimiter (\\t)")) -> ("new file path (Not A Path if cancelled)"=w449:path)  [unwired: 10 in, 1 out]
                    }
                    frame #2 {
                      n269 = call-poly <vilib>:"Write Delimited Spreadsheet.vi"("file path (dialog if empty)"=w466, "1D data"=string[] ["VD/V", "VG/V", "ID/A", "IS/A", "IG/A"], "append to file? (new file:F)"=TRUE, "delimiter (\\t)"="," ("delimiter (\\t)")) -> ("new file path (Not A Path if cancelled)"=w463:path)  [unwired: 10 in, 1 out]
                    }
                    frame #3 {
                      n270 = property on="VD OUTPUT" class="Arr (strict)"() -> ("Value"=w476:dbl[])  [unwired: 2 in, 2 out]
                      n271 = property on="ID OUTPUT" class="Arr (strict)"() -> ("Value"=w474:dbl[])  [unwired: 2 in, 2 out]
                      n272 = property on="IG OUTPUT" class="Arr (strict)"() -> ("Value"=w472:dbl[])  [unwired: 2 in, 2 out]
                      n273 = property on="VG OC MEA" class="Arr (strict)"() -> ("Value"=w475:dbl[])  [unwired: 2 in, 2 out]
                      n274 = property on="IS OUTPUT" class="Arr (strict)"() -> ("Value"=w473:dbl[])  [unwired: 2 in, 2 out]
                      n275 = Build Array(w476, w475, w474, w473, w472) -> (w471:dbl[][])
                      n276 = call-poly <vilib>:"Write Delimited Spreadsheet.vi"("file path (dialog if empty)"=w470, "format (%.3f)"="%.5e", "2D data"=w471, "append to file? (new file:F)"=TRUE, "transpose? (no:F)"=TRUE, "delimiter (\\t)"="," ("delimiter (\\t)")) -> ()  [unwired: 8 in, 2 out]
                    }
                  }
                }
              }
            }
            frame #7 {
            }
          }
          n277 = case shown="False" w281 {
            selector: w281 -> [_ w286]
            tunnel: [w285 w286] -> w283
            tunnel: w282 -> [w285 _]
            frame False {
            }
            frame True {
            }
          }
        }
      }
    }
  }
  n278 = while {
    stop <- FALSE stop-if-true
    n279 = event shown="[0] \"RUN OUTPUT\": Value Change" {
      selector: _ -> [_]
      dyn-events: _ -> [_]
      timeout: _ -> [_]
      event "RUN OUTPUT": Value Change {
        n280 = event-data() -> ()  [unwired: 1 in, 6 out]
        n281 = flat-sequence {
          frame #0 {
            n282 = property on="output number of times" class="DigNum (strict)"("Value"=0.0 ("output number of times")) -> ()  [unwired: 2 in, 2 out]
          }
          frame #1 {
            n283 = property on="Step for VDS [V] for OC" class="DigNum (strict)"() -> ("Value"=w485:dbl)  [unwired: 2 in, 2 out]
            n284 = property on="Maximum VDS [V] for OC" class="DigNum (strict)"() -> ("Value"=w486:dbl)  [unwired: 2 in, 2 out]
            n285 = invoke on="VDS" class="Arr (strict)" method="Reinit To Default"() -> ()  [unwired: 3 in, 3 out]
            n286 = invoke on="IDS 1" class="Arr (strict)" method="Reinit To Default"() -> ()  [unwired: 3 in, 3 out]
            n287 = invoke on="IDS 2" class="Arr (strict)" method="Reinit To Default"() -> ()  [unwired: 3 in, 3 out]
            n288 = invoke on="IDS 3" class="Arr (strict)" method="Reinit To Default"() -> ()  [unwired: 3 in, 3 out]
            n289 = invoke on="IDS 4" class="Arr (strict)" method="Reinit To Default"() -> ()  [unwired: 3 in, 3 out]
            n290 = invoke on="IDS 5" class="Arr (strict)" method="Reinit To Default"() -> ()  [unwired: 3 in, 3 out]
            n291 = invoke on="IDS 6" class="Arr (strict)" method="Reinit To Default"() -> ()  [unwired: 3 in, 3 out]
            n292 = Divide(x=w486, y=w485) -> (x/y=w484:dbl)
            n293 = Add(x=w484, y=1.0) -> (x+y=w482:dbl)
            n294 = property on="output TEM" class="DigNum (strict)"("Value"=0.0 ("output TEM")) -> ()  [unwired: 2 in, 2 out]
            n295 = property on="output number of times" class="DigNum (strict)"("Value"=w482) -> ()  [unwired: 2 in, 2 out]
            n296 = property on="state" class="DigNum (strict)"("Value"=0.0 ("state")) -> ()  [unwired: 2 in, 2 out]
          }
          frame #2 {
            n297 = property on="output number of times" class="DigNum (strict)"() -> ("Value"=w488:dbl)  [unwired: 2 in, 2 out]
            n298 = for {
              N: w488 -> [_]
              i -> [w490]
              n299 = property on="Step for VDS [V] for OC" class="DigNum (strict)"() -> ("Value"=w489:dbl)  [unwired: 2 in, 2 out]
              n300 = Greater Than 0?(x=w490) -> (x > 0?=w491:bool)
              n301 = case shown="True" w491 {
                tunnel: w490 -> [w494 w496]
                tunnel: w489 -> [_ w497]
                frame False {
                  n302 = property on="VDS" class="Arr (strict)"() -> ("Value"=w495:dbl[])  [unwired: 2 in, 2 out]
                  n303 = Insert Into Array(array=w495, index=w494, new element=0.0 ("new element/subarray")) -> (w493:dbl[])
                  n304 = property on="VDS" class="Arr (strict)"("Value"=w493) -> ()  [unwired: 2 in, 2 out]
                }
                frame True {
                  n305 = flat-sequence {
                    tunnel: w497 -> [w499]
                    tunnel: w496 -> [w503]
                    frame #0 {
                      n306 = property on="output TEM" class="DigNum (strict)"() -> ("Value"=w500:dbl)  [unwired: 2 in, 2 out]
                      n307 = Add(x=w499, y=w500) -> (x+y=w498:dbl)
                      n308 = property on="output TEM" class="DigNum (strict)"("Value"=w498) -> ()  [unwired: 2 in, 2 out]
                    }
                    frame #1 {
                      n309 = property on="output TEM" class="DigNum (strict)"() -> ("Value"=w502:dbl)  [unwired: 2 in, 2 out]
                      n310 = property on="VDS" class="Arr (strict)"() -> ("Value"=w504:dbl[])  [unwired: 2 in, 2 out]
                      n311 = Insert Into Array(array=w504, index=w503, new element=w502) -> (w501:dbl[])
                      n312 = property on="VDS" class="Arr (strict)"("Value"=w501) -> ()  [unwired: 2 in, 2 out]
                    }
                  }
                }
              }
            }
          }
          frame #3 {
            n313 = for {
              N: 6 -> [_]
              i -> [w506]
              n314 = case shown="0, Default" w506 {
                tunnel: [w671 w672 w673 w674 w675 w676] -> w507
                frame 0, Default {
                  n315 = property on="VGS[1] [V] for OC" class="DigNum (strict)"() -> ("Value"=w671:dbl)  [unwired: 2 in, 2 out]
                }
                frame 1 {
                  n316 = property on="VGS[2] [V] for OC" class="DigNum (strict)"() -> ("Value"=w672:dbl)  [unwired: 2 in, 2 out]
                }
                frame 2 {
                  n317 = property on="VGS[3] [V] for OC" class="DigNum (strict)"() -> ("Value"=w673:dbl)  [unwired: 2 in, 2 out]
                }
                frame 3 {
                  n318 = property on="VGS[4] [V] for OC" class="DigNum (strict)"() -> ("Value"=w674:dbl)  [unwired: 2 in, 2 out]
                }
                frame 4 {
                  n319 = property on="VGS[5] [V] for OC" class="DigNum (strict)"() -> ("Value"=w675:dbl)  [unwired: 2 in, 2 out]
                }
                frame 5 {
                  n320 = property on="VG[6] [V] for OC" class="DigNum (strict)"() -> ("Value"=w676:dbl)  [unwired: 2 in, 2 out]
                }
              }
              n321 = property on="output number of times" class="DigNum (strict)"() -> ("Value"=w508:dbl)  [unwired: 2 in, 2 out]
              n322 = for {
                N: w508 -> [_]
                tunnel: w507 -> [w510]
                tunnel: w506 -> [w513]
                i -> [w512]
                n323 = flat-sequence {
                  tunnel: w510 -> [w516]
                  tunnel: w510 -> [w523]
                  tunnel: w512 -> [w520]
                  tunnel: w510 -> [w519]
                  tunnel: w513 -> [w536]
                  tunnel: w512 -> [w535]
                  tunnel: w510 -> [w534]
                  frame #0 {
                    n324 = property on="VT [V] for OC" class="DigNum (strict)"() -> ("Value"=w515:dbl)  [unwired: 2 in, 2 out]
                    n325 = Less Or Equal?(x=w516, y=w515) -> (x <= y?=w514:bool)
                    n326 = case shown="True" w514 {
                      frame False {
                        n327 = property on="state" class="DigNum (strict)"("Value"=0.0 ("state")) -> ()  [unwired: 2 in, 2 out]
                      }
                      frame True {
                        n328 = property on="state" class="DigNum (strict)"("Value"=1.0 ("state")) -> ()  [unwired: 2 in, 2 out]
                      }
                    }
                  }
                  frame #1 {
                    n329 = property on="VT [V] for OC" class="DigNum (strict)"() -> ("Value"=w522:dbl)  [unwired: 2 in, 2 out]
                    n330 = Greater?(x=w523, y=w522) -> (0:w521:bool)
                    n331 = case shown="True" w521 {
                      tunnel: w520 -> [_ w530]
                      tunnel: w519 -> [_ w529]
                      frame False {
                        n332 = property on="state" class="DigNum (strict)"("Value"=1.0 ("state")) -> ()  [unwired: 2 in, 2 out]
                      }
                      frame True {
                        n333 = property on="VDS" class="Arr (strict)"() -> ("Value"=w531:dbl[])  [unwired: 2 in, 2 out]
                        n334 = Index Array(array=w531, index=w530) -> (element=w527:dbl)
                        n335 = property on="VT [V] for OC" class="DigNum (strict)"() -> ("Value"=w528:dbl)  [unwired: 2 in, 2 out]
                        n336 = Subtract(x=w529, y=w528) -> (x-y=w526:dbl)
                        n337 = Less Or Equal?(x=w527, y=w526) -> (x <= y?=w525:bool)
                        n338 = case shown="True" w525 {
                          frame False {
                            n339 = property on="state" class="DigNum (strict)"("Value"=3.0 ("state")) -> ()  [unwired: 2 in, 2 out]
                          }
                          frame True {
                            n340 = property on="state" class="DigNum (strict)"("Value"=2.0 ("state")) -> ()  [unwired: 2 in, 2 out]
                          }
                        }
                      }
                    }
                  }
                  frame #2 {
                    n341 = property on="state" class="DigNum (strict)"() -> ("Value"=w537:dbl)  [unwired: 2 in, 2 out]
                    n342 = case shown="1" w537 {
                      tunnel: w536 -> [_ w539 w566 w621]
                      tunnel: w535 -> [_ w538 w565 w620]
                      tunnel: w534 -> [_ _ w574 w626]
                      frame 0, Default {
                      }
                      frame 1 {
                        n343 = case shown="0, Default" w539 {
                          tunnel: w538 -> [w542 w547 w550 w554 w558 w562]
                          frame 0, Default {
                            n344 = property on="IDS 1" class="Arr (strict)"() -> ("Value"=w543:dbl[])  [unwired: 2 in, 2 out]
                            n345 = Insert Into Array(array=w543, index=w542, new element=0.0 ("new element/subarray")) -> (w540:dbl[])
                            n346 = property on="IDS 1" class="Arr (strict)"("Value"=w540) -> ()  [unwired: 2 in, 2 out]
                          }
                          frame 1 {
                            n347 = property on="IDS 2" class="Arr (strict)"() -> ("Value"=w546:dbl[])  [unwired: 2 in, 2 out]
                            n348 = Insert Into Array(array=w546, index=w547, new element=0.0 ("new element/subarray")) -> (w545:dbl[])
                            n349 = property on="IDS 2" class="Arr (strict)"("Value"=w545) -> ()  [unwired: 2 in, 2 out]
                          }
                          frame 2 {
                            n350 = property on="IDS 3" class="Arr (strict)"() -> ("Value"=w551:dbl[])  [unwired: 2 in, 2 out]
                            n351 = Insert Into Array(array=w551, index=w550, new element=0.0 ("new element/subarray")) -> (w548:dbl[])
                            n352 = property on="IDS 3" class="Arr (strict)"("Value"=w548) -> ()  [unwired: 2 in, 2 out]
                          }
                          frame 3 {
                            n353 = property on="IDS 4" class="Arr (strict)"() -> ("Value"=w555:dbl[])  [unwired: 2 in, 2 out]
                            n354 = Insert Into Array(array=w555, index=w554, new element=0.0 ("new element/subarray")) -> (w552:dbl[])
                            n355 = property on="IDS 4" class="Arr (strict)"("Value"=w552) -> ()  [unwired: 2 in, 2 out]
                          }
                          frame 4 {
                            n356 = property on="IDS 5" class="Arr (strict)"() -> ("Value"=w559:dbl[])  [unwired: 2 in, 2 out]
                            n357 = Insert Into Array(array=w559, index=w558, new element=0.0 ("new element/subarray")) -> (w556:dbl[])
                            n358 = property on="IDS 5" class="Arr (strict)"("Value"=w556) -> ()  [unwired: 2 in, 2 out]
                          }
                          frame 5 {
                            n359 = property on="IDS 6" class="Arr (strict)"() -> ("Value"=w563:dbl[])  [unwired: 2 in, 2 out]
                            n360 = Insert Into Array(array=w563, index=w562, new element=0.0 ("new element/subarray")) -> (w560:dbl[])
                            n361 = property on="IDS 6" class="Arr (strict)"("Value"=w560) -> ()  [unwired: 2 in, 2 out]
                          }
                        }
                      }
                      frame 2 {
                        n362 = property on="Transistor capacitance [nF/cm^2] for OC" class="DigNum (strict)"() -> ("Value"=w568:dbl)  [unwired: 2 in, 2 out]
                        n363 = property on="Transistor length [cm] for OC" class="DigNum (strict)"() -> ("Value"=w570:dbl)  [unwired: 2 in, 2 out]
                        n364 = property on="Predicted mobility [cm^2/Vs] for OC" class="DigNum (strict)"() -> ("Value"=w569:dbl)  [unwired: 2 in, 2 out]
                        n365 = property on="Transistor width [cm] for OC" class="DigNum (strict)"() -> ("Value"=w571:dbl)  [unwired: 2 in, 2 out]
                        n366 = property on="VDS" class="Arr (strict)"() -> ("Value"=w573:dbl[])  [unwired: 2 in, 2 out]
                        n367 = property on="VT [V] for OC" class="DigNum (strict)"() -> ("Value"=w567:dbl)  [unwired: 2 in, 2 out]
                        n368 = Index Array(array=w573, index=w565) -> (element=w572:dbl)
                        n369 = xnode "Formula"("W"=w571, "L"=w570, "u"=w569, "C"=w568, "VG"=w574, "VT"=w567, "VDS"=w572) -> ("Result"=w564:dbl)  [unwired: 1 in, 1 out]
                        n370 = case shown="5" w566 {
                          tunnel: w565 -> [w577 w582 w585 w589 w593 w597]
                          tunnel: w564 -> [w576 w580 w584 w588 w592 w596]
                          frame 0, Default {
                            n371 = property on="IDS 1" class="Arr (strict)"() -> ("Value"=w578:dbl[])  [unwired: 2 in, 2 out]
                            n372 = Insert Into Array(array=w578, index=w577, new element=w576) -> (w575:dbl[])
                            n373 = property on="IDS 1" class="Arr (strict)"("Value"=w575) -> ()  [unwired: 2 in, 2 out]
                          }
                          frame 1 {
                            n374 = property on="IDS 2" class="Arr (strict)"() -> ("Value"=w581:dbl[])  [unwired: 2 in, 2 out]
                            n375 = Insert Into Array(array=w581, index=w582, new element=w580) -> (w579:dbl[])
                            n376 = property on="IDS 2" class="Arr (strict)"("Value"=w579) -> ()  [unwired: 2 in, 2 out]
                          }
                          frame 2 {
                            n377 = property on="IDS 3" class="Arr (strict)"() -> ("Value"=w586:dbl[])  [unwired: 2 in, 2 out]
                            n378 = Insert Into Array(array=w586, index=w585, new element=w584) -> (w583:dbl[])
                            n379 = property on="IDS 3" class="Arr (strict)"("Value"=w583) -> ()  [unwired: 2 in, 2 out]
                          }
                          frame 3 {
                            n380 = property on="IDS 4" class="Arr (strict)"() -> ("Value"=w590:dbl[])  [unwired: 2 in, 2 out]
                            n381 = Insert Into Array(array=w590, index=w589, new element=w588) -> (w587:dbl[])
                            n382 = property on="IDS 4" class="Arr (strict)"("Value"=w587) -> ()  [unwired: 2 in, 2 out]
                          }
                          frame 4 {
                            n383 = property on="IDS 5" class="Arr (strict)"() -> ("Value"=w594:dbl[])  [unwired: 2 in, 2 out]
                            n384 = Insert Into Array(array=w594, index=w593, new element=w592) -> (w591:dbl[])
                            n385 = property on="IDS 5" class="Arr (strict)"("Value"=w591) -> ()  [unwired: 2 in, 2 out]
                          }
                          frame 5 {
                            n386 = property on="IDS 6" class="Arr (strict)"() -> ("Value"=w598:dbl[])  [unwired: 2 in, 2 out]
                            n387 = Insert Into Array(array=w598, index=w597, new element=w596) -> (w595:dbl[])
                            n388 = property on="IDS 6" class="Arr (strict)"("Value"=w595) -> ()  [unwired: 2 in, 2 out]
                          }
                        }
                      }
                      frame 3 {
                        n389 = property on="Transistor capacitance [nF/cm^2] for OC" class="DigNum (strict)"() -> ("Value"=w627:dbl)  [unwired: 2 in, 2 out]
                        n390 = property on="Transistor length [cm] for OC" class="DigNum (strict)"() -> ("Value"=w623:dbl)  [unwired: 2 in, 2 out]
                        n391 = property on="Predicted mobility [cm^2/Vs] for OC" class="DigNum (strict)"() -> ("Value"=w624:dbl)  [unwired: 2 in, 2 out]
                        n392 = property on="VT [V] for OC" class="DigNum (strict)"() -> ("Value"=w625:dbl)  [unwired: 2 in, 2 out]
                        n393 = property on="Transistor width [cm] for OC" class="DigNum (strict)"() -> ("Value"=w622:dbl)  [unwired: 2 in, 2 out]
                        n394 = xnode "Formula"("W"=w622, "L"=w623, "u"=w624, "C"=w627, "VG"=w626, "VT"=w625) -> ("Result"=w619:dbl)  [unwired: 1 in, 1 out]
                        n395 = case shown="5" w621 {
                          tunnel: w620 -> [w630 w634 w638 w642 w646 w650]
                          tunnel: w619 -> [w629 w633 w637 w641 w645 w649]
                          frame 0, Default {
                            n396 = property on="IDS 1" class="Arr (strict)"() -> ("Value"=w631:dbl[])  [unwired: 2 in, 2 out]
                            n397 = Insert Into Array(array=w631, index=w630, new element=w629) -> (w628:dbl[])
                            n398 = property on="IDS 1" class="Arr (strict)"("Value"=w628) -> ()  [unwired: 2 in, 2 out]
                          }
                          frame 1 {
                            n399 = property on="IDS 2" class="Arr (strict)"() -> ("Value"=w635:dbl[])  [unwired: 2 in, 2 out]
                            n400 = Insert Into Array(array=w635, index=w634, new element=w633) -> (w632:dbl[])
                            n401 = property on="IDS 2" class="Arr (strict)"("Value"=w632) -> ()  [unwired: 2 in, 2 out]
                          }
                          frame 2 {
                            n402 = property on="IDS 3" class="Arr (strict)"() -> ("Value"=w639:dbl[])  [unwired: 2 in, 2 out]
                            n403 = Insert Into Array(array=w639, index=w638, new element=w637) -> (w636:dbl[])
                            n404 = property on="IDS 3" class="Arr (strict)"("Value"=w636) -> ()  [unwired: 2 in, 2 out]
                          }
                          frame 3 {
                            n405 = property on="IDS 4" class="Arr (strict)"() -> ("Value"=w643:dbl[])  [unwired: 2 in, 2 out]
                            n406 = Insert Into Array(array=w643, index=w642, new element=w641) -> (w640:dbl[])
                            n407 = property on="IDS 4" class="Arr (strict)"("Value"=w640) -> ()  [unwired: 2 in, 2 out]
                          }
                          frame 4 {
                            n408 = property on="IDS 5" class="Arr (strict)"() -> ("Value"=w647:dbl[])  [unwired: 2 in, 2 out]
                            n409 = Insert Into Array(array=w647, index=w646, new element=w645) -> (w644:dbl[])
                            n410 = property on="IDS 5" class="Arr (strict)"("Value"=w644) -> ()  [unwired: 2 in, 2 out]
                          }
                          frame 5 {
                            n411 = property on="IDS 6" class="Arr (strict)"() -> ("Value"=w651:dbl[])  [unwired: 2 in, 2 out]
                            n412 = Insert Into Array(array=w651, index=w650, new element=w649) -> (w648:dbl[])
                            n413 = property on="IDS 6" class="Arr (strict)"("Value"=w648) -> ()  [unwired: 2 in, 2 out]
                          }
                        }
                      }
                    }
                  }
                  frame #3 {
                    n414 = property on="state" class="DigNum (strict)"("Value"=0.0 ("state")) -> ()  [unwired: 2 in, 2 out]
                  }
                }
                n415 = Build Array (concatenate)("SIM VG OUT", w510) -> (w509:dbl[])
                n416 = property on="SIM VG OUT" class="Arr (strict)"("Value"=w509) -> ()  [unwired: 2 in, 2 out]
              }
            }
          }
          frame #4 {
            n417 = property on="IDS 1" class="Arr (strict)"() -> ("Value"=w690:dbl[])  [unwired: 2 in, 2 out]
            n418 = property on="IDS 2" class="Arr (strict)"() -> ("Value"=w688:dbl[])  [unwired: 2 in, 2 out]
            n419 = property on="IDS 3" class="Arr (strict)"() -> ("Value"=w686:dbl[])  [unwired: 2 in, 2 out]
            n420 = property on="IDS 4" class="Arr (strict)"() -> ("Value"=w684:dbl[])  [unwired: 2 in, 2 out]
            n421 = property on="IDS 5" class="Arr (strict)"() -> ("Value"=w682:dbl[])  [unwired: 2 in, 2 out]
            n422 = property on="IDS 6" class="Arr (strict)"() -> ("Value"=w681:dbl[])  [unwired: 2 in, 2 out]
            n423 = property on="VDS" class="Arr (strict)"() -> ("Value"=w683:dbl[])  [unwired: 2 in, 2 out]
            n424 = Bundle("Value"=w683, "Value"=w690) -> (w689:cluster{"Value":dbl[], "Value":dbl[]})  [unwired: 1 in]
            n425 = Bundle("Value"=w683, "Value"=w684) -> (w680:cluster{"Value":dbl[], "Value":dbl[]})  [unwired: 1 in]
            n426 = Bundle("Value"=w683, "Value"=w686) -> (w685:cluster{"Value":dbl[], "Value":dbl[]})  [unwired: 1 in]
            n427 = Bundle("Value"=w683, "Value"=w688) -> (w687:cluster{"Value":dbl[], "Value":dbl[]})  [unwired: 1 in]
            n428 = Bundle("Value"=w683, "Value"=w682) -> (w679:cluster{"Value":dbl[], "Value":dbl[]})  [unwired: 1 in]
            n429 = Bundle("Value"=w683, "Value"=w681) -> (w678:cluster{"Value":dbl[], "Value":dbl[]})  [unwired: 1 in]
            n430 = Build Array(w689, w687, w685, w680, w679, w678) -> (→"Output characteristic simulation":cluster{"Value":dbl[], "Value":dbl[]}[])
          }
          frame #5 {
            n431 = Two Button Dialog(message="Do you want to save data? (If save, please save as .csv)", 1:"Don't save" ("F button name (\"Cancel\")"), 2:"Save" ("T button name (\"OK\")")) -> (T button?=w691:bool)
            n432 = case shown="True" w691 {
              frame False {
              }
              frame True {
                n433 = flat-sequence {
                  tunnel: [w703] -> w698
                  tunnel: [w710] -> w697
                  tunnel: w698 -> [w705]
                  tunnel: w697 -> [w715]
                  tunnel: [w714] -> w695
                  tunnel: [w725] -> w696
                  tunnel: w695 -> [w726]
                  tunnel: [w730] -> w699
                  tunnel: w696 -> [w728]
                  tunnel: w699 -> [w744]
                  frame #0 {
                    n434 = call-poly <vilib>:"Write Delimited Spreadsheet.vi"("1D data"=string[] ["Date", "Time"], "append to file? (new file:F)"=TRUE, "delimiter (\\t)"="," ("delimiter (\\t)")) -> ("new file path (Not A Path if cancelled)"=w703:path)  [unwired: 11 in, 1 out]
                  }
                  frame #1 {
                    n435 = Get Date/Time String() -> (date string=w709:string, time string=w708:string)  [unwired: 3 in]
                    n436 = Build Array(w709, w708) -> (w707:string[])
                    n437 = call-poly <vilib>:"Write Delimited Spreadsheet.vi"("file path (dialog if empty)"=w705, "1D data"=w707, "append to file? (new file:F)"=TRUE, "delimiter (\\t)"="," ("delimiter (\\t)")) -> ("new file path (Not A Path if cancelled)"=w710:path)  [unwired: 10 in, 1 out]
                  }
                  frame #2 {
                    n438 = call-poly <vilib>:"Write Delimited Spreadsheet.vi"("file path (dialog if empty)"=w715, "1D data"=string[] ["VG1/V", "VG2/V", "VG3/V", "VG4/V", "VG5/V", "VG6/V"], "append to file? (new file:F)"=TRUE, "delimiter (\\t)"="," ("delimiter (\\t)")) -> ("new file path (Not A Path if cancelled)"=w714:path)  [unwired: 10 in, 1 out]
                  }
                  frame #3 {
                    n439 = property on="VGS[2] [V] for OC" class="DigNum (strict)"() -> ("Value"=w722:dbl)  [unwired: 2 in, 2 out]
                    n440 = property on="VGS[1] [V] for OC" class="DigNum (strict)"() -> ("Value"=w723:dbl)  [unwired: 2 in, 2 out]
                    n441 = property on="VGS[3] [V] for OC" class="DigNum (strict)"() -> ("Value"=w721:dbl)  [unwired: 2 in, 2 out]
                    n442 = property on="VGS[5] [V] for OC" class="DigNum (strict)"() -> ("Value"=w719:dbl)  [unwired: 2 in, 2 out]
                    n443 = property on="VGS[4] [V] for OC" class="DigNum (strict)"() -> ("Value"=w720:dbl)  [unwired: 2 in, 2 out]
                    n444 = property on="VG[6] [V] for OC" class="DigNum (strict)"() -> ("Value"=w718:dbl)  [unwired: 2 in, 2 out]
                    n445 = Build Array(w723, w722, w721, w720, w719, w718) -> (w716:dbl[])
                    n446 = call-poly <vilib>:"Write Delimited Spreadsheet.vi"("file path (dialog if empty)"=w726, "1D data"=w716, "append to file? (new file:F)"=TRUE, "delimiter (\\t)"="," ("delimiter (\\t)")) -> ("new file path (Not A Path if cancelled)"=w725:path)  [unwired: 10 in, 1 out]
                  }
                  frame #4 {
                    n447 = call-poly <vilib>:"Write Delimited Spreadsheet.vi"("file path (dialog if empty)"=w728, "1D data"=string[] ["VDS/V", "IDS1/A", "IDS2/A", "IDS3/A", "IDS4/A", "IDS5/A", "IDS6/A", ""], "append to file? (new file:F)"=TRUE, "delimiter (\\t)"="," ("delimiter (\\t)")) -> ("new file path (Not A Path if cancelled)"=w730:path)  [unwired: 10 in, 1 out]
                  }
                  frame #5 {
                    n448 = property on="VDS" class="Arr (strict)"() -> ("Value"=w743:dbl[])  [unwired: 2 in, 2 out]
                    n449 = property on="IDS 1" class="Arr (strict)"() -> ("Value"=w737:dbl[])  [unwired: 2 in, 2 out]
                    n450 = property on="IDS 2" class="Arr (strict)"() -> ("Value"=w736:dbl[])  [unwired: 2 in, 2 out]
                    n451 = property on="IDS 3" class="Arr (strict)"() -> ("Value"=w735:dbl[])  [unwired: 2 in, 2 out]
                    n452 = property on="IDS 4" class="Arr (strict)"() -> ("Value"=w734:dbl[])  [unwired: 2 in, 2 out]
                    n453 = property on="IDS 6" class="Arr (strict)"() -> ("Value"=w732:dbl[])  [unwired: 2 in, 2 out]
                    n454 = property on="IDS 5" class="Arr (strict)"() -> ("Value"=w733:dbl[])  [unwired: 2 in, 2 out]
                    n455 = Build Array(w743, w737, w736, w735, w734, w733, w732) -> (w742:dbl[][])
                    n456 = call-poly <vilib>:"Write Delimited Spreadsheet.vi"("file path (dialog if empty)"=w744, "format (%.3f)"="%.5e", "2D data"=w742, "append to file? (new file:F)"=TRUE, "transpose? (no:F)"=TRUE, "delimiter (\\t)"="," ("delimiter (\\t)")) -> ()  [unwired: 8 in, 2 out]
                  }
                }
              }
            }
          }
        }
      }
    }
  }
  n457 = while {
    stop <- FALSE stop-if-true
    (unwired) enum32{"Output", " Transfer", "Simulation"}."Output" ("Tab Control")
    n458 = event shown="[0] \"run\": Value Change" {
      selector: _ -> [_]
      dyn-events: _ -> [_]
      timeout: _ -> [_]
      event "run": Value Change {
        n459 = event-data() -> ()  [unwired: 1 in, 6 out]
        n460 = flat-sequence {
          frame #0 {
            n461 = property on="transfer number of times" class="DigNum (strict)"("Value"=0.0 ("number of times")) -> ()  [unwired: 2 in, 2 out]
          }
          frame #1 {
            n462 = property on="Step for VGS [V] for TC" class="DigNum (strict)"() -> ("Value"=w750:dbl)  [unwired: 2 in, 2 out]
            n463 = property on="VGS [V] for TC" class="DigNum (strict)"() -> ("Value"=w751:dbl)  [unwired: 2 in, 2 out]
            n464 = invoke on="IDS" class="Arr (strict)" method="Reinit To Default"() -> ()  [unwired: 3 in, 3 out]
            n465 = invoke on="VG" class="Arr (strict)" method="Reinit To Default"() -> ()  [unwired: 3 in, 3 out]
            n466 = property on="transfer Tem" class="DigNum (strict)"("Value"=0.0 ("Tem")) -> ()  [unwired: 2 in, 2 out]
            n467 = Divide(x=w751, y=w750) -> (x/y=w749:dbl)
            n468 = Add(x=w749, y=1.0) -> (x+y=w747:dbl)
            n469 = property on="transfer number of times" class="DigNum (strict)"("Value"=w747) -> ()  [unwired: 2 in, 2 out]
          }
          frame #2 {
            n470 = property on="transfer number of times" class="DigNum (strict)"() -> ("Value"=w753:dbl)  [unwired: 2 in, 2 out]
            n471 = for {
              N: w753 -> [_]
              i -> [w756]
              n472 = property on="Step for VGS [V] for TC" class="DigNum (strict)"() -> ("Value"=w754:dbl)  [unwired: 2 in, 2 out]
              n473 = Greater Than 0?(x=w756) -> (x > 0?=w755:bool)
              n474 = case shown="True" w755 {
                tunnel: w756 -> [w759 w761]
                tunnel: w754 -> [_ w762]
                frame False {
                  n475 = property on="VG" class="Arr (strict)"() -> ("Value"=w758:dbl[])  [unwired: 2 in, 2 out]
                  n476 = Insert Into Array(array=w758, index=w759, new element=0.0 ("new element/subarray")) -> (w757:dbl[])
                  n477 = property on="VG" class="Arr (strict)"("Value"=w757) -> ()  [unwired: 2 in, 2 out]
                }
                frame True {
                  n478 = flat-sequence {
                    tunnel: w762 -> [w765]
                    tunnel: w761 -> [w769]
                    frame #0 {
                      n479 = property on="transfer Tem" class="DigNum (strict)"() -> ("Value"=w764:dbl)  [unwired: 2 in, 2 out]
                      n480 = Add(x=w765, y=w764) -> (x+y=w763:dbl)
                      n481 = property on="transfer Tem" class="DigNum (strict)"("Value"=w763) -> ()  [unwired: 2 in, 2 out]
                    }
                    frame #1 {
                      n482 = property on="VG" class="Arr (strict)"() -> ("Value"=w768:dbl[])  [unwired: 2 in, 2 out]
                      n483 = property on="transfer Tem" class="DigNum (strict)"() -> ("Value"=w766:dbl)  [unwired: 2 in, 2 out]
                      n484 = Insert Into Array(array=w768, index=w769, new element=w766) -> (w767:dbl[])
                      n485 = property on="VG" class="Arr (strict)"("Value"=w767) -> ()  [unwired: 2 in, 2 out]
                    }
                  }
                }
              }
            }
          }
          frame #3 {
            n486 = property on="transfer number of times" class="DigNum (strict)"() -> ("Value"=w770:dbl)  [unwired: 2 in, 2 out]
            n487 = for {
              N: w770 -> [_]
              i -> [w771]
              n488 = flat-sequence {
                tunnel: w771 -> [w777]
                frame #0 {
                  n489 = property on="VG" class="Arr (strict)"() -> ("Value"=w773:dbl[])  [unwired: 2 in, 2 out]
                  n490 = Index Array(array=w773, index=w777) -> (element=w778:dbl)
                  n491 = property on="VT [V] for TC" class="DigNum (strict)"() -> ("Value"=w772:dbl)  [unwired: 2 in, 2 out]
                  n492 = Subtract(x=w778, y=w772) -> (x-y=w775:dbl)
                  n493 = Less Or Equal To 0?(x=w775) -> (x <= 0?=w776:bool)
                  n494 = case shown="True" w776 {
                    tunnel: w777 -> [w786 w797]
                    tunnel: [w785 w796] -> w774
                    tunnel: w775 -> [w784 w794]
                    frame False {
                      n495 = property on="Transistor length [cm] for TC" class="DigNum (strict)"() -> ("Value"=w779:dbl)  [unwired: 2 in, 2 out]
                      n496 = property on="Predicted mobility [cm^2/Vs] for TC" class="DigNum (strict)"() -> ("Value"=w781:dbl)  [unwired: 2 in, 2 out]
                      n497 = property on="Transistor width [cm] for TC" class="DigNum (strict)"() -> ("Value"=w783:dbl)  [unwired: 2 in, 2 out]
                      n498 = property on="Transistor capacitance [nF/cm^2] for TC" class="DigNum (strict)"() -> ("Value"=w782:dbl)  [unwired: 2 in, 2 out]
                      n499 = Divide(x=w783, y=w779) -> (x/y=w791:dbl)
                      n500 = Multiply(x=w782, y=w791) -> (x*y=w790:dbl)
                      n501 = Square(x=w784) -> (x^2=w788:dbl)
                      n502 = Multiply(x=w790, y=w781) -> (x*y=w789:dbl)
                      n503 = Multiply(x=w789, y=w788) -> (x*y=w787:dbl)
                      n504 = property on="IDS" class="Arr (strict)"() -> ("Value"=w780:dbl[])  [unwired: 2 in, 2 out]
                      n505 = Insert Into Array(array=w780, index=w786, new element=w787) -> (w785:dbl[])
                    }
                    frame True {
                      n506 = Multiply(x=0.0, y=w794) -> (x*y=w793:dbl)
                      n507 = property on="IDS" class="Arr (strict)"() -> ("Value"=w792:dbl[])  [unwired: 2 in, 2 out]
                      n508 = Insert Into Array(array=w792, index=w797, new element=w793) -> (w796:dbl[])
                    }
                  }
                  n509 = property on="IDS" class="Arr (strict)"("Value"=w774) -> ()  [unwired: 2 in, 2 out]
                }
              }
            }
          }
          frame #4 {
            n510 = property on="VG" class="Arr (strict)"() -> ("Value"=w800:dbl[])  [unwired: 2 in, 2 out]
            n511 = property on="IDS" class="Arr (strict)"() -> ("Value"=w799:dbl[])  [unwired: 2 in, 2 out]
            n512 = call "Convert to Dynamic Data2"("Array"=w800) -> ("Dynamic Data Type"=w802:dynamicdata)  [unwired: 3 in]
            n513 = call "Convert to Dynamic Data"("Array"=w799) -> ("Dynamic Data Type"=w801:dynamicdata)  [unwired: 3 in]
            n514 = call "Build XY Graph"("Y Input"=w801, "X Input"=w802) -> ("XY Graph"=→"Transfer characteristic simulation":cluster{"Y":dbl[], "Y":dbl[]}[])  [unwired: 3 in, 6 out]
          }
          frame #5 {
            n515 = Two Button Dialog(message="Do you want to save data? (If save, please save as .csv)", 1:"Don't save" ("F button name (\"Cancel\")"), 2:"Save" ("T button name (\"OK\")")) -> (T button?=w803:bool)
            n516 = case shown="True" w803 {
              frame False {
              }
              frame True {
                n517 = flat-sequence {
                  tunnel: [w810] -> w809
                  tunnel: w809 -> [w818]
                  tunnel: [w817] -> w808
                  tunnel: w808 -> [w825]
                  tunnel: [w824] -> w807
                  tunnel: w807 -> [w826]
                  frame #0 {
                    n518 = call-poly <vilib>:"Write Delimited Spreadsheet.vi"("1D data"=string[] ["Date", "Time"], "append to file? (new file:F)"=TRUE, "delimiter (\\t)"="," ("delimiter (\\t)")) -> ("new file path (Not A Path if cancelled)"=w810:path)  [unwired: 11 in, 1 out]
                  }
                  frame #1 {
                    n519 = Get Date/Time String() -> (date string=w816:string, time string=w815:string)  [unwired: 3 in]
                    n520 = Build Array(w816, w815) -> (w814:string[])
                    n521 = call-poly <vilib>:"Write Delimited Spreadsheet.vi"("file path (dialog if empty)"=w818, "1D data"=w814, "append to file? (new file:F)"=TRUE, "delimiter (\\t)"="," ("delimiter (\\t)")) -> ("new file path (Not A Path if cancelled)"=w817:path)  [unwired: 10 in, 1 out]
                  }
                  frame #2 {
                    n522 = call-poly <vilib>:"Write Delimited Spreadsheet.vi"("file path (dialog if empty)"=w825, "1D data"=string[] ["VG/V", "IDS/A"], "append to file? (new file:F)"=TRUE, "delimiter (\\t)"="," ("delimiter (\\t)")) -> ("new file path (Not A Path if cancelled)"=w824:path)  [unwired: 10 in, 1 out]
                  }
                  frame #3 {
                    n523 = property on="VG" class="Arr (strict)"() -> ("Value"=w832:dbl[])  [unwired: 2 in, 2 out]
                    n524 = property on="IDS" class="Arr (strict)"() -> ("Value"=w831:dbl[])  [unwired: 2 in, 2 out]
                    n525 = Build Array(w832, w831) -> (w833:dbl[][])
                    n526 = call-poly <vilib>:"Write Delimited Spreadsheet.vi"("file path (dialog if empty)"=w826, "format (%.3f)"="%.5e", "2D data"=w833, "append to file? (new file:F)"=TRUE, "transpose? (no:F)"=TRUE, "delimiter (\\t)"="," ("delimiter (\\t)")) -> ()  [unwired: 8 in, 2 out]
                  }
                }
              }
            }
          }
        }
      }
    }
  }
  n527 = while {
    stop <- FALSE stop-if-true
    n528 = event shown="[1] \"Clear\": Value Change" {
      selector: _ -> [_ _]
      dyn-events: _ -> [_ _]
      timeout: _ -> [_ _]
      event Timeout {
        n529 = event-data() -> ()  [unwired: 1 in, 3 out]
      }
      event "Clear": Value Change {
        n530 = event-data() -> ()  [unwired: 1 in, 6 out]
        n531 = flat-sequence {
          frame #0 {
            n532 = invoke on="VDS" class="Arr (strict)" method="Reinit To Default"() -> ()  [unwired: 3 in, 3 out]
            n533 = invoke on="IDS 1" class="Arr (strict)" method="Reinit To Default"() -> ()  [unwired: 3 in, 3 out]
            n534 = invoke on="IDS 3" class="Arr (strict)" method="Reinit To Default"() -> ()  [unwired: 3 in, 3 out]
            n535 = invoke on="IDS 4" class="Arr (strict)" method="Reinit To Default"() -> ()  [unwired: 3 in, 3 out]
            n536 = invoke on="IDS 2" class="Arr (strict)" method="Reinit To Default"() -> ()  [unwired: 3 in, 3 out]
            n537 = invoke on="IDS 5" class="Arr (strict)" method="Reinit To Default"() -> ()  [unwired: 3 in, 3 out]
            n538 = invoke on="VG" class="Arr (strict)" method="Reinit To Default"() -> ()  [unwired: 3 in, 3 out]
            n539 = invoke on="IDS" class="Arr (strict)" method="Reinit To Default"() -> ()  [unwired: 3 in, 3 out]
            n540 = invoke on="IDS 6" class="Arr (strict)" method="Reinit To Default"() -> ()  [unwired: 3 in, 3 out]
          }
          frame #1 {
            n541 = property on="VG" class="Arr (strict)"() -> ("Value"=w853:dbl[])  [unwired: 2 in, 2 out]
            n542 = property on="IDS" class="Arr (strict)"() -> ("Value"=w851:dbl[])  [unwired: 2 in, 2 out]
            n543 = call "Convert to Dynamic Data3"("Array"=w853) -> ("Dynamic Data Type"=w852:dynamicdata)  [unwired: 3 in]
            n544 = call "Convert to Dynamic Data4"("Array"=w851) -> ("Dynamic Data Type"=w850:dynamicdata)  [unwired: 3 in]
            n545 = call "Build XY Graph2"("Y Input"=w850, "X Input"=w852) -> ("XY Graph"=w849:cluster{"Y":dbl[], "Y":dbl[]}[])  [unwired: 3 in, 6 out]
            n546 = property on="IDS 5" class="Arr (strict)"() -> ("Value"=w842:dbl[])  [unwired: 2 in, 2 out]
            n547 = property on="Transfer characteristic simulation" class="XYGraph (strict)"("Value"=w849) -> ()  [unwired: 2 in, 2 out]
            n548 = property on="IDS 6" class="Arr (strict)"() -> ("Value"=w841:dbl[])  [unwired: 2 in, 2 out]
            n549 = property on="IDS 4" class="Arr (strict)"() -> ("Value"=w843:dbl[])  [unwired: 2 in, 2 out]
            n550 = property on="VDS" class="Arr (strict)"() -> ("Value"=w844:dbl[])  [unwired: 2 in, 2 out]
            n551 = property on="IDS 3" class="Arr (strict)"() -> ("Value"=w845:dbl[])  [unwired: 2 in, 2 out]
            n552 = property on="IDS 1" class="Arr (strict)"() -> ("Value"=w848:dbl[])  [unwired: 2 in, 2 out]
            n553 = property on="IDS 2" class="Arr (strict)"() -> ("Value"=w846:dbl[])  [unwired: 2 in, 2 out]
            n554 = Bundle("Value"=w844, "Value"=w848) -> (w847:cluster{"Value":dbl[], "Value":dbl[]})  [unwired: 1 in]
            n555 = Bundle("Value"=w844, "Value"=w842) -> (w837:cluster{"Value":dbl[], "Value":dbl[]})  [unwired: 1 in]
            n556 = Bundle("Value"=w844, "Value"=w841) -> (w836:cluster{"Value":dbl[], "Value":dbl[]})  [unwired: 1 in]
            n557 = Bundle("Value"=w844, "Value"=w845) -> (w839:cluster{"Value":dbl[], "Value":dbl[]})  [unwired: 1 in]
            n558 = Bundle("Value"=w844, "Value"=w846) -> (w840:cluster{"Value":dbl[], "Value":dbl[]})  [unwired: 1 in]
            n559 = Bundle("Value"=w844, "Value"=w843) -> (w838:cluster{"Value":dbl[], "Value":dbl[]})  [unwired: 1 in]
            n560 = Build Array(w847, w840, w839, w838, w837, w836) -> (w835:cluster{"Value":dbl[], "Value":dbl[]}[])
            n561 = property on="Output characteristic simulation" class="XYGraph (strict)"("Value"=w835) -> ()  [unwired: 2 in, 2 out]
          }
        }
      }
    }
  }
